vi "WSVCAP SHL FPGA TL Top Level.vi"() -> ()   [LabVIEW 2012]
uses:
  Type Defs/WSVCAP SHL State.ctl
  Type Defs/WSVCAP SHL Transaction Enum.ctl
  Type Defs/WSVCAP SHL Communication Loop State.ctl
  Type Defs/WSVCAP SHL FIFO Operation Enum.ctl
  Type Defs/WSVCAP SHL Operation Step Enum.ctl
  Type Defs/WSVCAP SHL Procedure Step Enum.ctl
  Type Defs/WSVCAP SHL Transaction Step Enum.ctl
  <vilib>/Platform/TimedLoop/XDataNode/timing_clust.ctl
  <vilib>/Platform/TimedLoop/XDataNode/nitl_modes.ctl
  <vilib>/Platform/TimedLoop/XDataNode/wakeup.ctl
  WSVCAP Shell FPGA Low Level/WSVCAP SHL FPGA LL RFFE Debug Global.vi
  WSVCAP Shell FPGA Low Level/WSVCAP SHL FPGA LL SPI Debug Global.vi
  WSVCAP Shell FPGA Low Level/WSVCAP SHL FPGA LL I2C Debug Global.vi
  <vilib>/Platform/TimedLoop/XDataNode/XDataNode.xnode
  <vilib>/Platform/TimedLoop/XDataNode/XDNodeRunTimeDep.lvlib
panel:
  in  "Stop Cycle":bool
  out "Cycle Count":u64
  in  "Socket Mask":u64=1 format="%012x"
  in  "Display CH (1-48)":i32=1 min=1 max=48 step=1
  out "Status":i32
  out "Read Data":u64
  in  "Transaction":T1
  in  "Bytes to Write":u8=8
  in  "Sub Address":u8=1 format="%02x"
  in  "Ack Read Status":bool
  out "Read Status Flag":bool
  in  "Exit":bool
  out "Waveform Chart":cluster{i16, i16, i16, i16}(graph)
  in  "Wait Ticks":u32=20
  in  "Slave Address":u8=1 format="%02x"
  in  "Bytes to Read":u8=8
  in  "Start":bool
  in  "Cmd":T2
  in  "Ack Read":bool
  out "Read Flag":bool
  in  "Write Flag":bool
  in  "Write Data":u64
  # "Control"
  # "I2C Configuration Parameters"
  # "Host Data Transfer"
  # "Command Type"
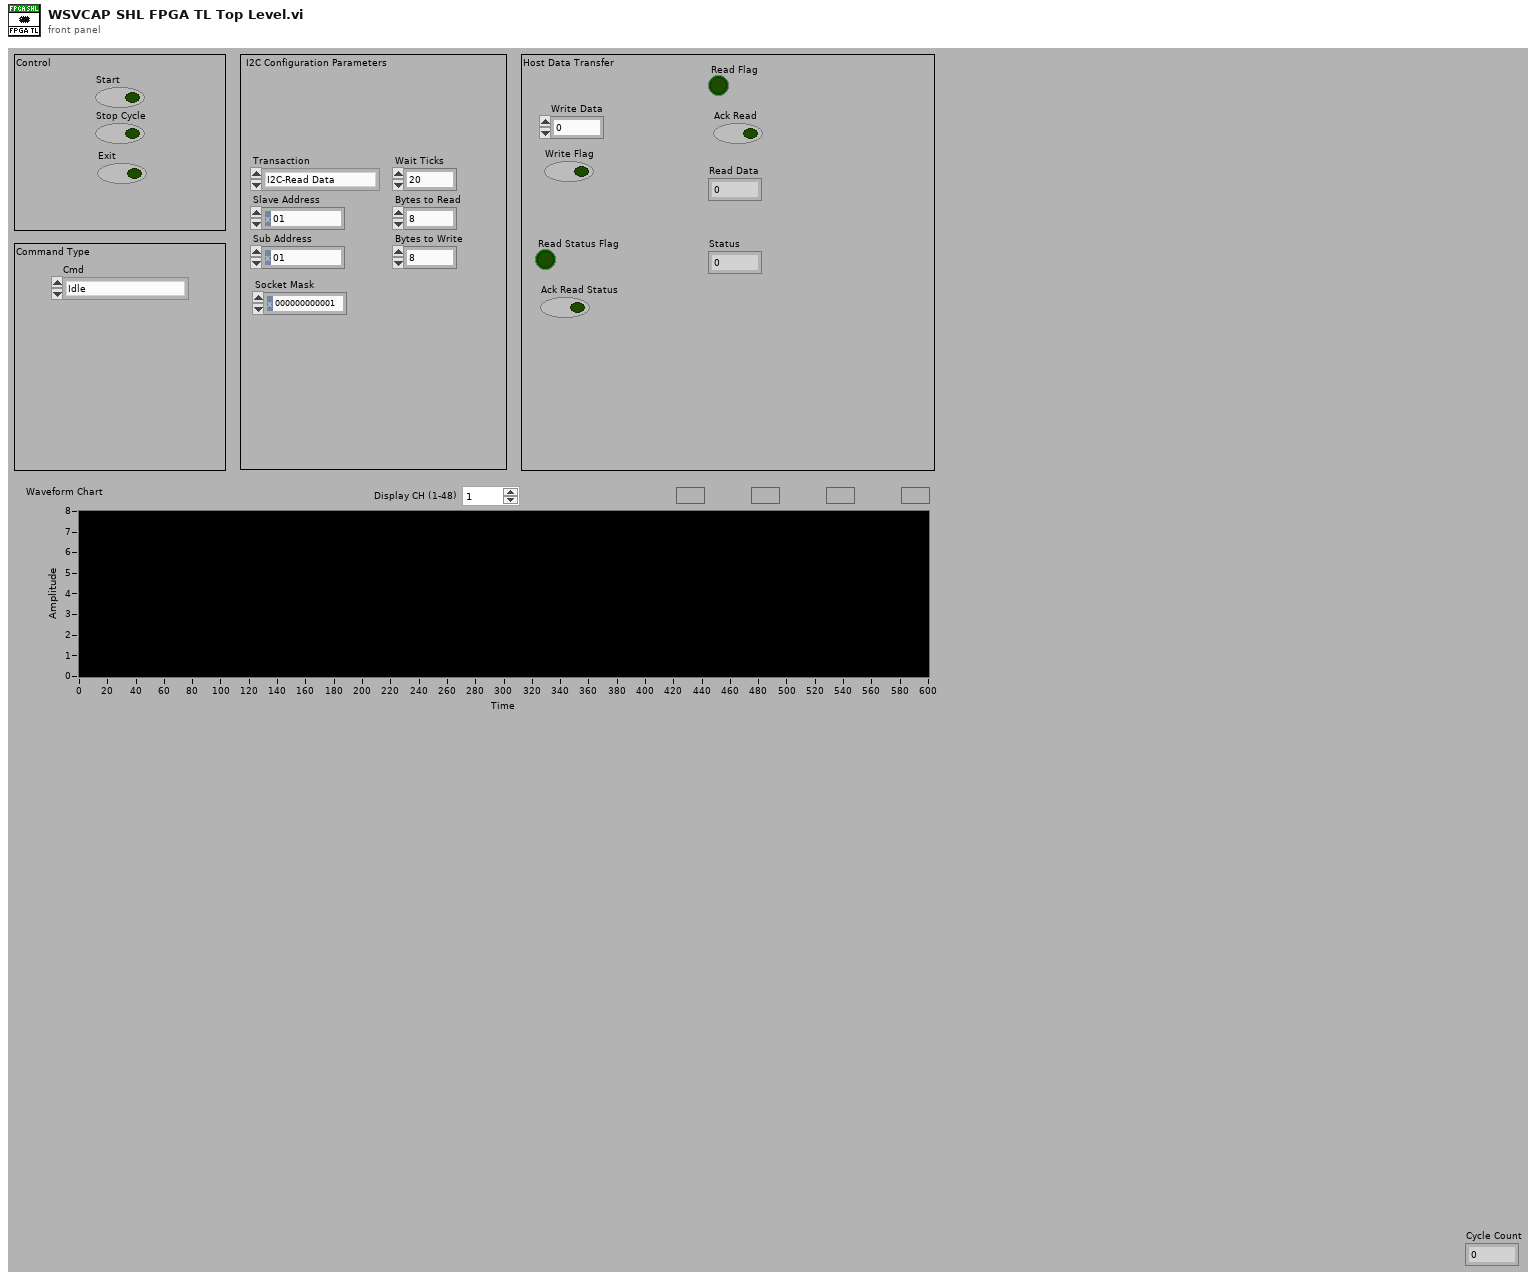
[diagram p1: front panel]
types:
  T1 = typedef "WSVCAP SHL Transaction Enum.ctl" = enum16{"I2C-Read Data", "I2C-Write Data", "SPI-Write/Read Data", "RFFE-Ext Write", "RFFE-Ext Read"}
  T2 = typedef "WSVCAP SHL State.ctl" = enum8{"Idle", "Transfer Data"}
  T3 = typedef "WSVCAP SHL Communication Loop State.ctl" = enum8{"Idle", "Initialize", "Pre-Transmission", "Transmit Data", "Post Transmition", "Operation Complete"}
  T4 = typedef "WSVCAP SHL FIFO Operation Enum.ctl" = enum16{"Create FIFO/Memory", "Get Write FIFO Status", "Get Read FIFO Status", "Put Element in Write", "Put Element in Read", "Get Element from Write", "Get Element from Read"}
  T5 = typedef "WSVCAP SHL Procedure Step Enum.ctl" = enum16{"I2C Start/Stop - 1: Set Clock Low", "I2C Start/Stop - 2: Wait", "I2C Start/Stop - 3: Set Data I", "I2C Start/Stop - 4: Wait", "I2C Start/Stop - 5: Set Clock High", "I2C Start/Stop - 6: Wait", "I2C Start/Stop - 7: Set Data II", "I2C Start/Stop - 8: Wait", "I2C Start/Stop - 9: Set Clock Low", "I2C Start/Stop - 10: Wait", "I2C Read ACK - 1: Set Clock High", "I2C Read ACK - 2: Wait", "I2C Read ACK - 3: Read ACK Bit", "I2C Read ACK - 4: Wait", "I2C Read ACK - 5: Set Clock Low", "I2C Read ACK - 6: Wait", "I2C Write ACK - 1: Write ACK Bit", "I2C Write ACK - 2: Wait", "I2C Write ACK - 3: Set Clock High", "I2C Write ACK - 4: Wait", "I2C Write ACK - 5: Set Clock Low", "I2C Write ACK - 6: Wait", "I2C Write ACK - 7: Set Data Low", "I2C Send Add - 1: Reset Bits Remaining", "I2C Send Add - 2: Set Data Bit", "I2C Send Add - 3: Wait", "I2C Send Add - 4: Set Clock High", "I2C Send Add - 5: Wait", "I2C Send Add - 6: Set Clock Low", "I2C Send Add - 7: Wait", "I2C Send Add - 8: Check Bits Remaining", "I2C Send Data - 1: Reset Bits Remaining", "I2C Send Data - 2: Load Write Bit from FIFO", "I2C Send Data - 3: Set Data Bit", "I2C Send Data - 4: Wait", "I2C Send Data - 5: Set Clock High", "I2C Send Data - 6: Wait", "I2C Send Data - 7: Set Clock Low", "I2C Send Data - 8: Wait", "I2C Send Data - 9: Check Bits Remaining", "I2C Receive Data - 1: Reset Bits Remaining", "I2C Receive Data - 2: Wait", "I2C Receive Data - 3: Set Clock High", "I2C Receive Data - 4: Wait", "I2C Receive Data - 5: Read Data Bit", "I2C Receive Data - 6: Wait", "I2C Receive Data - 7: Set Clock Low", "I2C Receive Data - 8: Wait", "I2C Receive Data - 9: Check Bits Remaining", "SPI Clear Lines - 1:Clear", "SPI Send/Receive - 1: Load SDA - Clock Low", "SPI Send/Receive - 2: Wait", "SPI Send/Receive - 3: Load DATO - Clock High", "SPI Send/Receive - 4: Wait", "SPI Wait CMD Delay - 1:Wait", "RFFE Send SSC - 1:Set Low", "RFFE Send SSC - 2:Wait", "RFFE Send SSC - 3:Set SDA High", "RFFE Send SSC - 4:Wait", "RFFE Send SSC - 5:Set SDA Low", "RFFE Send SSC - 6:Wait", "RFFE Send Data - 1:Set SCL High", "RFFE Send Data - 2:Wait", "RFFE Send Data - 3:Set SCL Low", "RFFE Send Data - 4:Wait", "RFFE Send Data - 5:Set SCL High (P)", "RFFE Send Data - 6:Wait", "RFFE Send Data - 7:Set SCL Low (P)", "RFFE Send Data - 8:Wait", "RFFE Send Data - 9:Set SCL High (BP)", "RFFE Send Data - 10:Wait", "RFFE Send Data - 11:Set SCL Low (BP)", "RFFE Send Data - 12:Wait", "RFFE Receive Data - 1:Set SCL High", "RFFE Receive Data - 2:Wait", "RFFE Receive Data - 3:Set SCL Low", "RFFE Receive Data - 4:Wait", "RFFE Receive Data - 5:Set SCL High (BP)", "RFFE Receive Data - 6:Wait", "RFFE Receive Data - 7:Set SCL Low (BP)", "RFFE Receive Data - 8:Wait", "RFFE Wait CMD Delay - 1:Wait", "RFFE Clear Lines - 1:Clear"}
  T6 = typedef "WSVCAP SHL Operation Step Enum.ctl" = enum16{"I2C Send Slave Add - A: Send Start Sequence", "I2C Send Slave Add - B: Load Address Byte", "I2C Send Slave Add - C: Send Address Byte", "I2C Send Slave Add - D: Read Slave ACK", "I2C Send Sub Add - A: Load Sub Address", "I2C Send Sub Add - B: Send Address Byte", "I2C Send Sub Add - C: Read Slave ACK", "I2C Send Data - A: Get Byte from FIFO", "I2C Send Data - B: Send Data Byte", "I2C Send Data - C: Read Slave ACK", "I2C Send Data - D: Send Stop Sequence", "I2C Read Data - A: Load Bytes to Read", "I2C Read Data - B: Receive Byte", "I2C Read Data - C: Write Master ACK", "I2C Read Data - D: Send Stop Sequence", "SPI Write/Read - A: SPI-Clear Lines", "SPI Write/Read - B: SPI-Send/Receive Data", "SPI Write/Read - C: SPI-Wait CMD Delay", "SPI Write/Read - D:SPI-Clear Lines", "RFFE Read Data - A: Send SSC", "RFFE Read Data - B: Send CMD Frame", "RFFE Read Data - C: Receive Byte", "RFFE Write Data - A: Send SSC", "RFFE Write Data - B: Send Data", "RFFE Write Data - C: Wait CMD Delay", "RFFE Write Data - D: Clear Lines"}
  T7 = typedef "WSVCAP SHL Transaction Step Enum.ctl" = enum16{"I2C Write - I:Send Slave Address", "I2C Write - II:Send Sub Address", "I2C Write - III:Send Data Bytes", "I2C Read - I:Send Slave Address (W)", "I2C Read - II:Send Sub Address", "I2C Read - III:Send Slave Address (R)", "I2C Read - IV:Read Data Bytes", "SPI Write/Read - I:SPI-Write/Read Data", "RFFE Ext Write - I.Write Data", "RFFE Ext Read - I:Read Data"}
  T8 = typedef "XDNodeRunTimeDep.lvlib/timing_clust.ctl" = cluster{"Expected End [f-1]":u64, "Actual End [f-1]":u64, "Finished Late? [f-1]":bool, "Expected End [i-1]":u64, "Actual End [i-1]":u64, "Finished Late? [i-1]":bool, "Expected Start [i]":u64, "Actual Start [i]":u64, "Expected Start [f]":u64, "Actual Start [f]":u64, "Source Name":string, "Structure Name":string, "Period":i64, "Deadline":i64, "Offset":i64, "Start":i64, "Priority":i32, "Timeout":i32, "Mode":T9, "Wakeup Reason":T10, "Error":errorcluster, "Source Type":string, "Secondary Source Type":string, "Global End Time":u64, "Global Start Time":u64, "Frame Duration":u64, "Iteration Duration":u64, "Assigned CPU":i32, "I/O Scan Engine Mode":u32}
  T9 = typedef "XDNodeRunTimeDep.lvlib/nitl_modes.ctl" = enum32{"No Change", "Process missed periods, maintain original phase", "Discard missed periods, maintain original phase", "Process missed periods, ignore original phase", "Discard missed periods, ignore original phase"}
  T10 = typedef "XDNodeRunTimeDep.lvlib/wakeup.ctl" = enum32{"Normal", "Aborted", "Asynchronous wakeup", "Timing source error", "Timed loop error", "Timeout"}
  T11 = typedef "WSVCAP SHL Transaction Cluster.ctl" = cluster{"Transaction":T1, "Write Byte":u8, "Write Bits Remaining":u8, "Read Bits Remaining":u8, "Read Bytes Remaining":u8, "Wait Ticks Remaining":u32, "Slave Address":u8, "Bytes to Read":u8, "Bytes to Write":u8, "Sub Address":u8, "Socket Mask":u64, "Write CMD [1-4]":u8, "Write Bit Index [0-39]":u8, "CMD Delay (Ticks)":u32, "Commands per Cycle [1-4]":u8, "CMD Length [1-48]":u8, "Cycle Count":u64, "Cycle Mode":bool, "CMD 1 Length (Bits)":u8, "CMD 2 Length (Bits)":u8, "CMD 3 Length (Bits)":u8, "CMD 4 Length (Bits)":u8, "CMD 1 Delay (Ticks)":u32, "CMD 2 Delay (Ticks)":u32, "CMD 3 Delay (Ticks)":u32, "CMD 4 Delay (Ticks)":u32, "CMD 1":u64, "CMD 2":u64, "CMD 3":u64, "CMD 4":u64, "Cycle CMD":u64, "Transaction Step":T7, "Operation Step":T6, "Procedure Step":T5, "Start Operation":bool, "Start Procedure":bool, "Procedure":T12, "Wait Ticks":u32}
  T12 = typedef "WSVCAP SHL Procedure Enum.ctl" = enum16{"None", "I2C-Send Start/Stop Sequence", "I2C-Send Address Byte", "I2C-Send Data Byte", "I2C-Read ACK", "I2C-Receive Byte", "I2C-Write ACK", "SPI-Clear Lines", "SPI-Send/Receive", "SPI-Wait CMD Delay", "RFFE-Clear Lines", "RFFE-Send SSC", "RFFE-Send Data", "RFFE-Receive Data", "RFFE-Wait CMD Delay"}
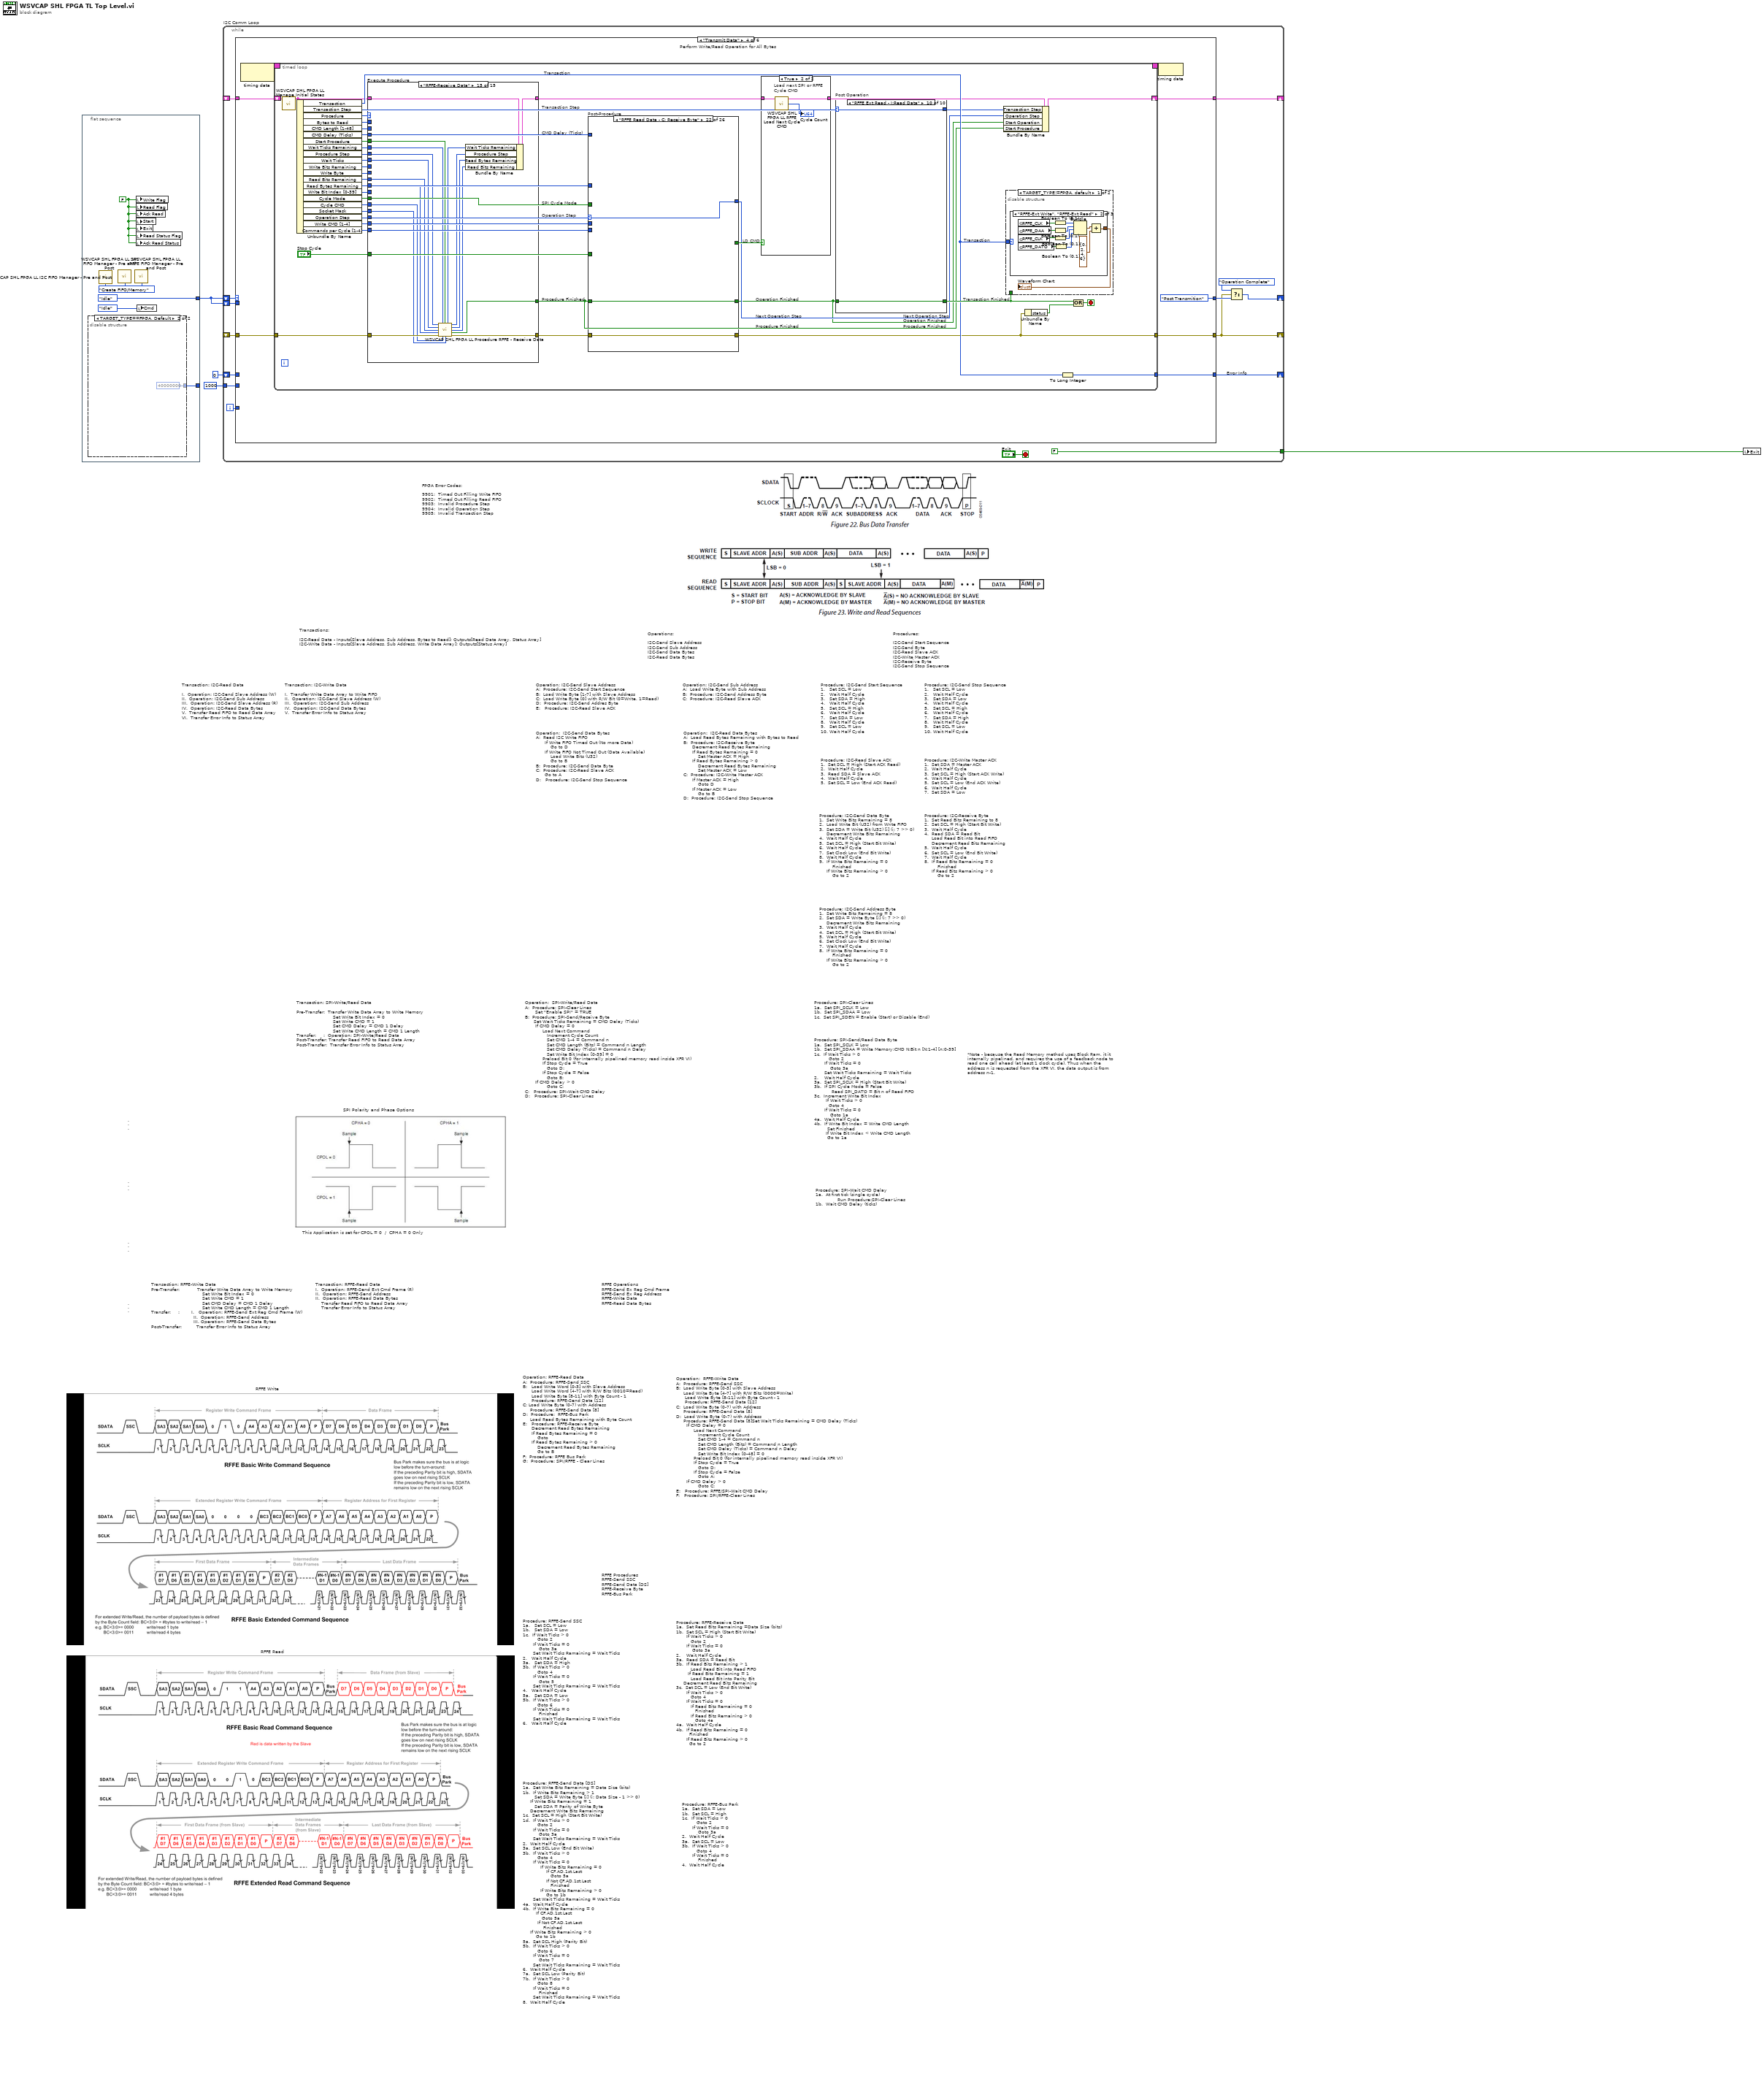
[diagram p0: block diagram]
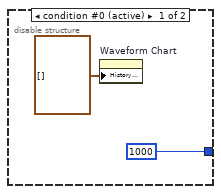
[diagram p2: hidden frame]
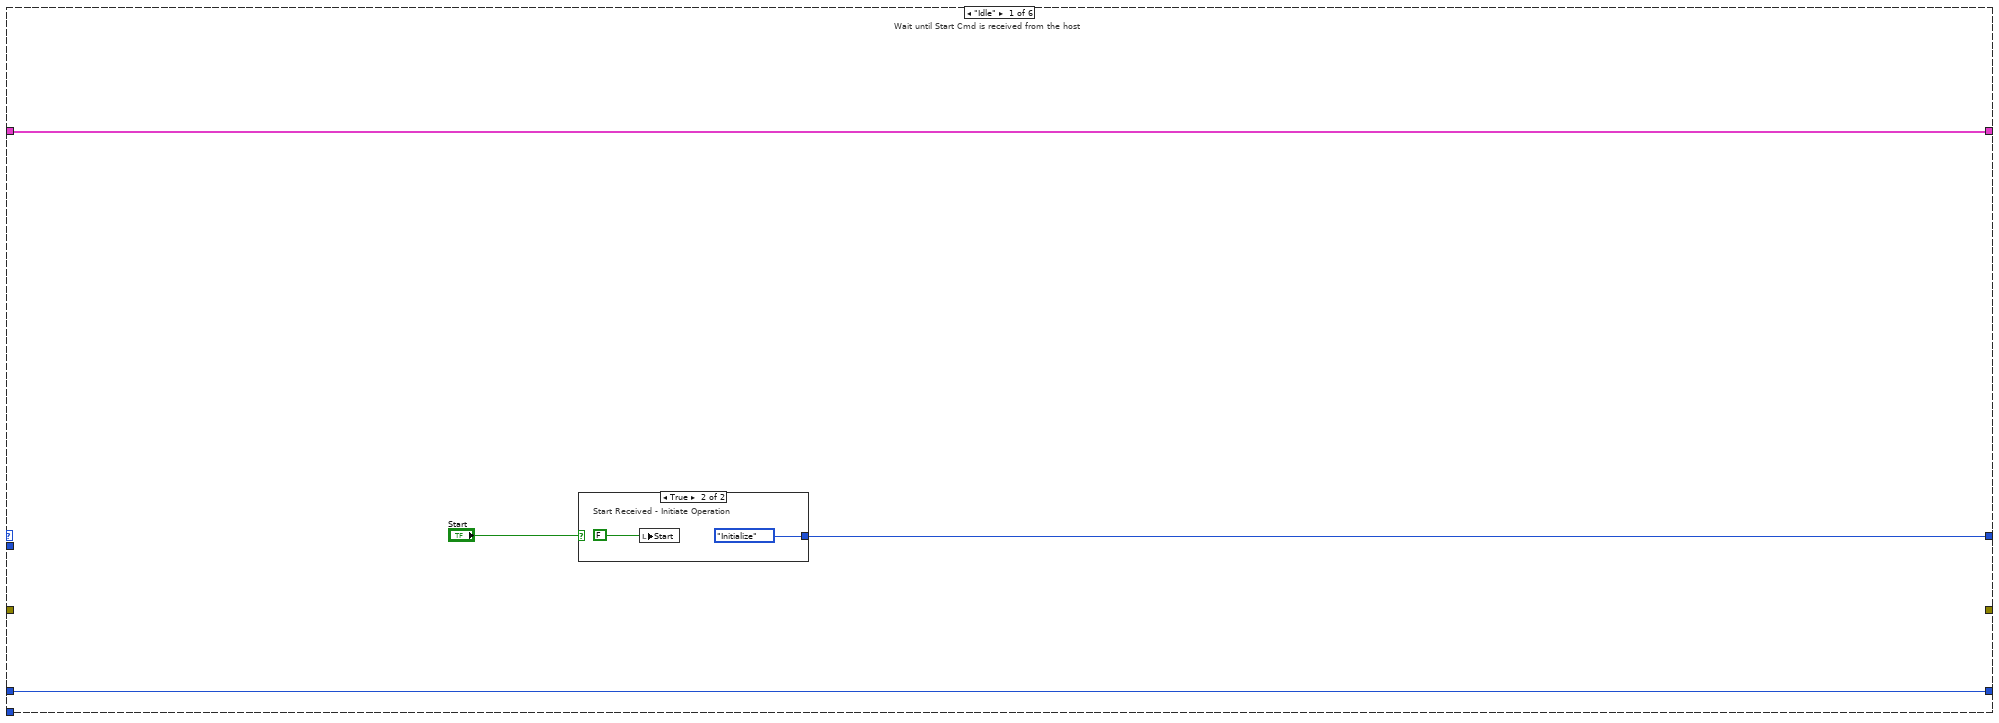
[diagram p3: hidden frame]
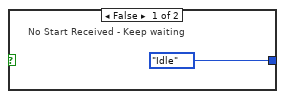
[diagram p4: hidden frame]
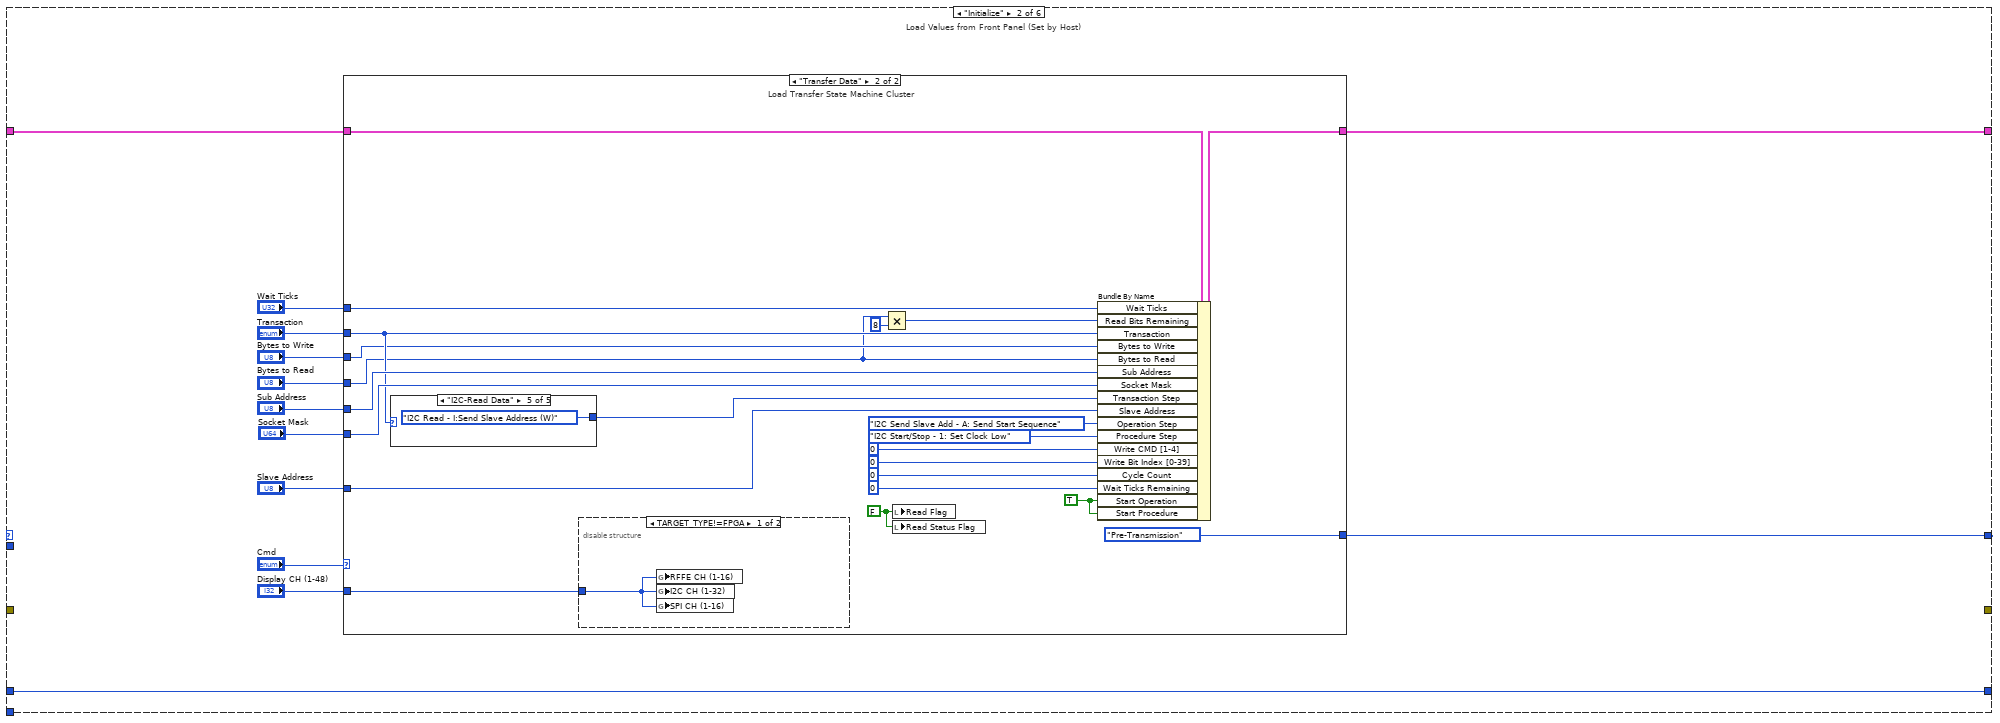
[diagram p5: hidden frame]
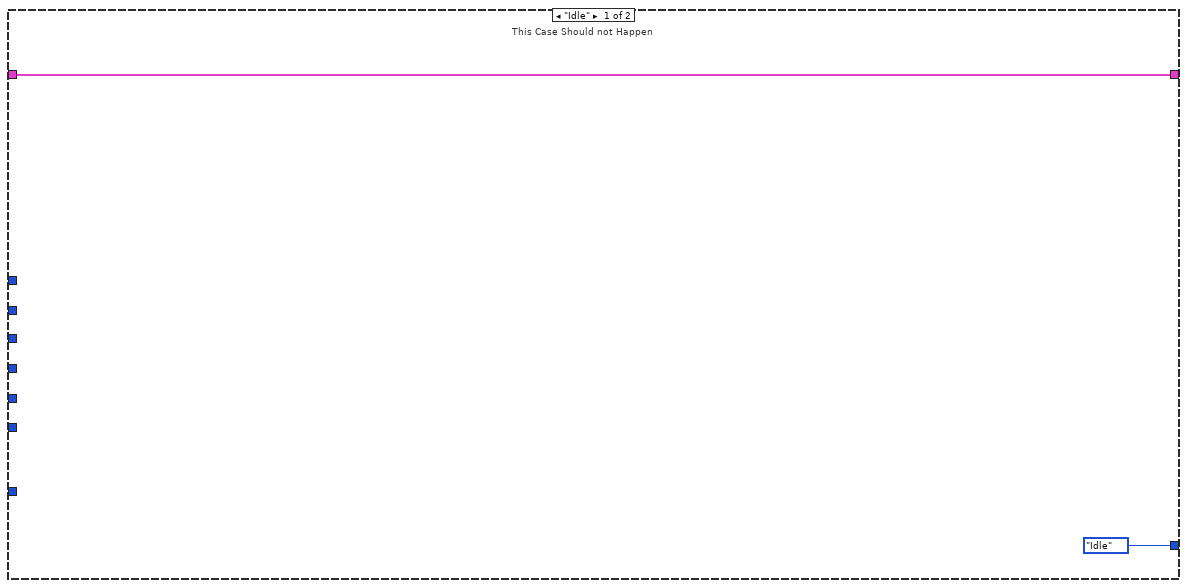
[diagram p6: hidden frame]
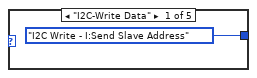
[diagram p7: hidden frame]
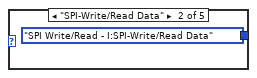
[diagram p8: hidden frame]
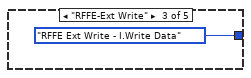
[diagram p9: hidden frame]
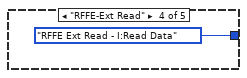
[diagram p10: hidden frame]
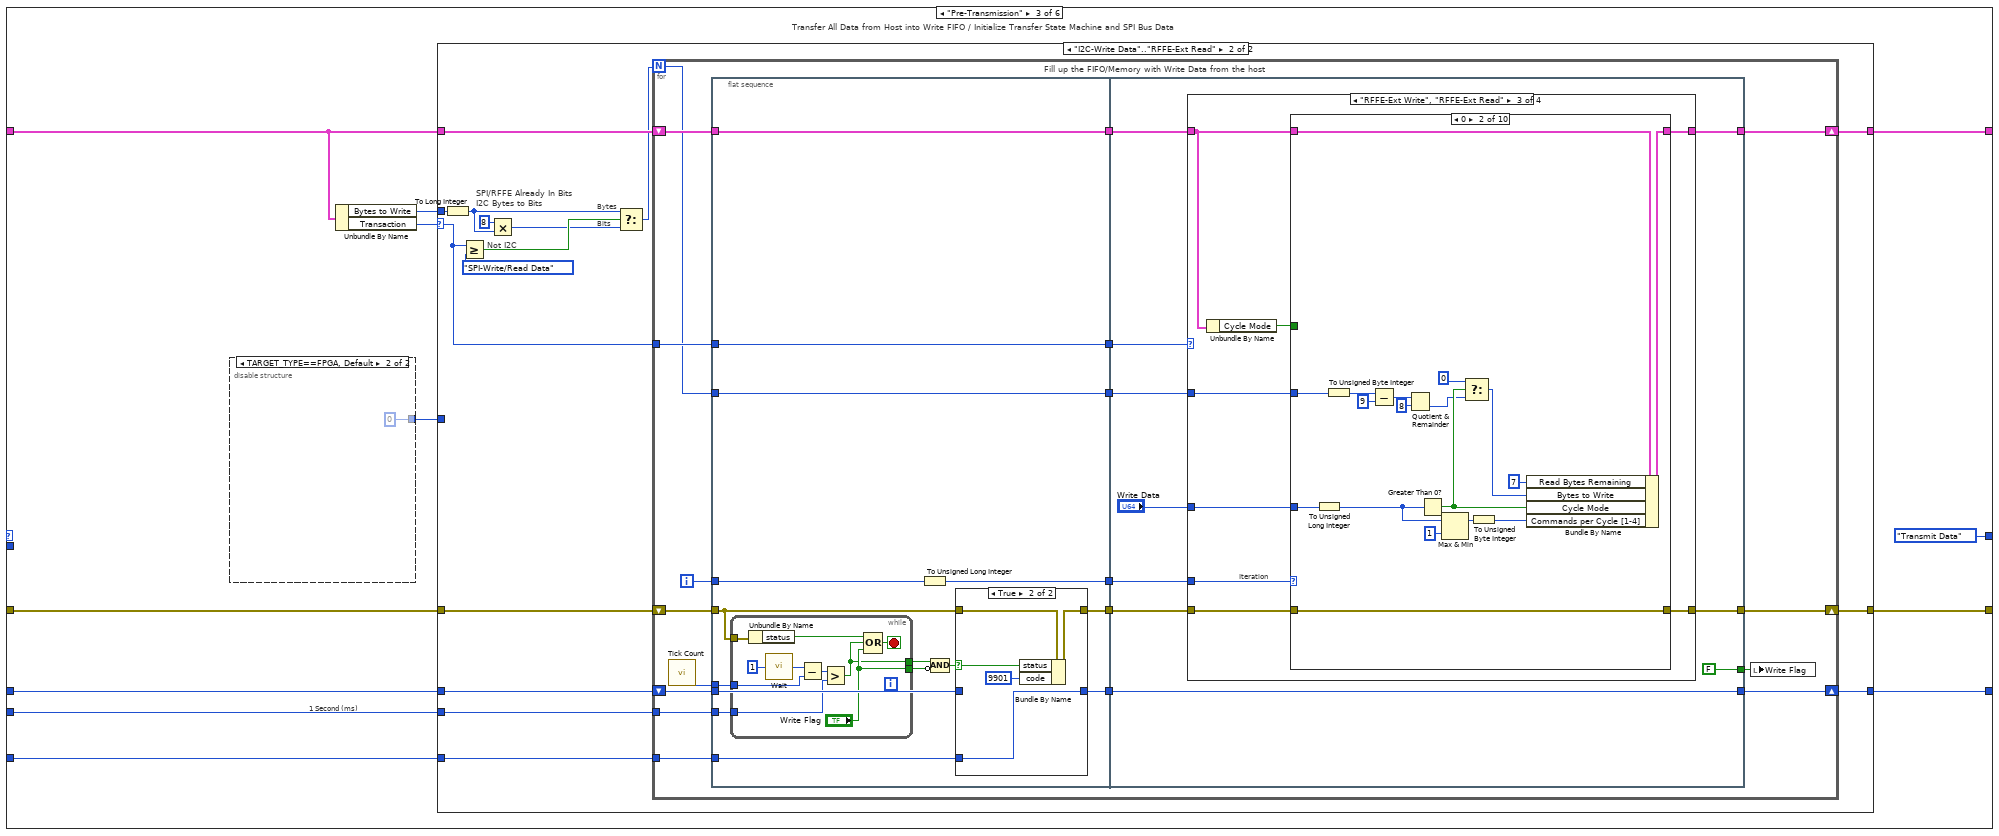
[diagram p12: hidden frame]
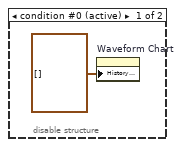
[diagram p13: hidden frame]
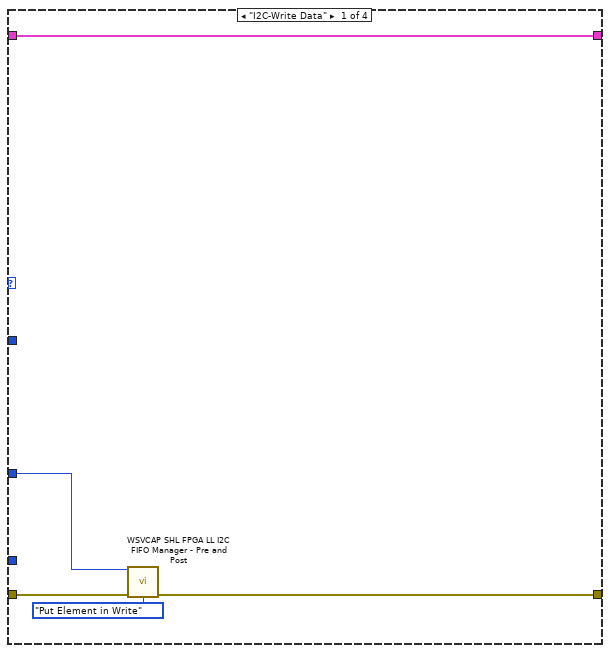
[diagram p16: hidden frame]
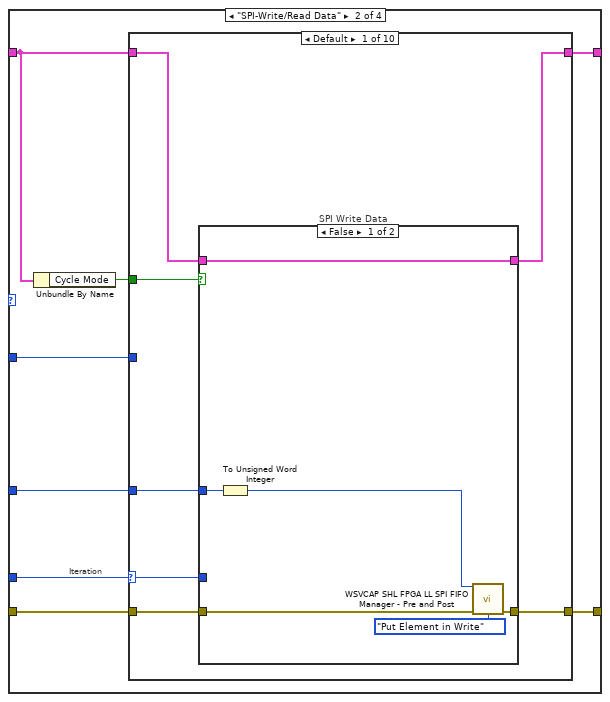
[diagram p17: hidden frame]
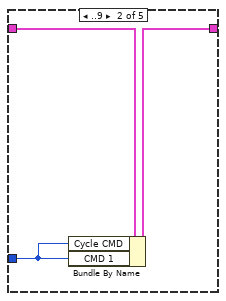
[diagram p19: hidden frame]
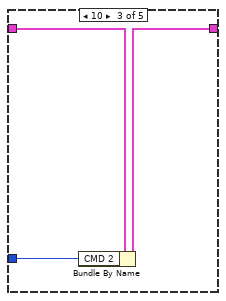
[diagram p20: hidden frame]
diagram:
  # "Operation:  RFFE-Write Data\nA:  Procedure: RFFE-Send SSC\nB:  Load Write Byte [0-3] with Slave Address\n     Load Write Byte [4-7] with R/W Bits (0000=Write)\n      Load Write Byte [8-11] with Byte Count - 1\n      Procedure: RFFE-Send Data [12]\nC:  Load Write Byte (0-7) with Address\n     Procedure: RFFE-Send Data [8]\nD:  Load Write Byte (0-7) with Address\n     Procedure: RFFE-Send Data [8]Set Wait Ticks Remaining = CMD Delay (Ticks)\n       If CMD Delay = 0\n            Load Next Command\n               Increment Cycle Count\n               Set CMD 1-4 = Command n\n               Set CMD Length (Bits) = Command n Length\n               Set CMD Delay (Ticks) = Command n Delay\n               Set Write Bit Index [0-48] = 0\n            Preload Bit 0 (for internally pipelined memory read inside XFR VI)\n            If Stop Cycle = True\n               Goto D:\n            If Stop Cycle = False\n               Goto A:\n       If CMD Delay > 0\n               Goto C:\nE:   Procedure: RFFE/SPI-Wait CMD Delay          \nF:   Procedure: SPI/RFFE-Clear Lines"
  # "Operation: RFFE-Read Data\nA:  Procedure: RFFE-Send SSC\nB:   Load Write Word [0-3] with Slave Address\n      Load Write Word [4-7] with R/W Bits (0010=Read)\n      Load Write Byte [8-11] with Byte Count - 1\n      Procedure: RFFE-Send Data [12]\nC: Load Write Byte (0-7) with Address\n     Procedure: RFFE-Send Data [8]\nD:  Procedure:  RFFE-Bus Park\n     Load Read Bytes Remaining with Byte Count\nE:   Procedure: RFFE-Receive Byte\n      Decrement Read Bytes Remaining\n      If Read Bytes Remaining = 0\n          Goto\n      If Read Bytes Remaining > 0\n          Decrement Read Bytes Remaining\n          Go to B\nF:  Procedure: RFFE Bus Park\nG:  Procedure: SPI/RFFE - Clear Lines"
  # "RFFE Write"
  # "RFFE Read"
  # "Transaction: RFFE-Write Data\nPre-Transfer:            Transfer Write Data Array to Write Memory\n                                   Set Write Bit Index = 0\n                                   Set Write CMD = 1\n                                   Set CMD Delay = CMD 1 Delay\n                                   Set Write CMD Length = CMD 1 Length\nTransfer:     :        I.   Operation: RFFE-Send Ext Reg Cmd Frame (W)\n                             II.  Operation: RFFE-Send Address\n                             III. Operation: RFFE-Send Data Bytes\nPost-Transfer:          Transfer Error Info to Status Array"
  # "Procedure: RFFE-Send Data [DS]\n1a.  Set Write Bits Remaining = Data Size (bits)\n1b.  If Write Bits Remaining > 1\n        Set SDA = Write Byte [i] (i: Data Size - 1 >> 0)\n     If Write Bits Remaining = 1\n        Set SDA = Parity of Write Byte\n     Decrement Write Bits Remaining\n1c.  Set SCL = High (Start Bit Write)\n1d.  If Wait Ticks > 0\n          Goto 2\n       If Wait Ticks = 0 \n           Goto 3a\n       Set Wait Ticks Ramaining = Wait Ticks\n2.  Wait Half Cycle\n3a.  Set SCL Low (End Bit Write)\n3b.  If Wait Ticks > 0\n          Goto 4\n       If Wait Ticks = 0 \n            If Write Bits Remaining = 0\n                If CF,AD,1st,Last\n                   Goto 5a\n                If Not CF,AD,1st,Last\n                   Finished\n            If Write Bits Remaining > 0\n                Go to 1b\n       Set Wait Ticks Ramaining = Wait Ticks\n4a.  Wait Half Cycle\n4b.  If Write Bits Remaining = 0\n         If CF,AD,1st,Last\n             Goto 5a\n          If Not CF,AD,1st,Last\n              Finished\n     If Write Bits Remaining > 0\n         Go to 1b\n5a.  Set SCL High (Parity Bit)\n5b.  If Wait Ticks > 0\n          Goto 6\n       If Wait Ticks = 0 \n           Goto 7\n       Set Wait Ticks Ramaining = Wait Ticks\n6.  Wait Half Cycle\n7a.  Set SCL Low (Parity Bit)\n7b.  If Wait Ticks > 0\n          Goto 8\n       If Wait Ticks = 0 \n           Finished\n       Set Wait Ticks Ramaining = Wait Ticks\n8.  Wait Half Cycle"
  # "Procedure: RFFE-Bus Park\n1a.  Set SDA = Low\n1b.  Set SCL = High\n1c.  If Wait Ticks > 0\n          Goto 2\n       If Wait Ticks = 0 \n           Goto 3a\n2.  Wait Half Cycle\n3a.  Set SCL = Low\n3b.  If Wait Ticks > 0\n          Goto 4\n       If Wait Ticks = 0 \n           Finished\n4.  Wait Half Cycle"
  # "Procedure: RFFE-Send SSC\n1a.   Set SCL = Low\n1b.   Set SDA = Low\n1c.  If Wait Ticks > 0\n          Goto 2\n       If Wait Ticks = 0 \n           Goto 3a\n       Set Wait Ticks Ramaining = Wait Ticks\n2.   Wait Half Cycle\n3a.   Set SDA = High\n3b.  If Wait Ticks > 0\n          Goto 4\n       If Wait Ticks = 0 \n           Goto 5\n       Set Wait Ticks Ramaining = Wait Ticks\n4.   Wait Half Cycle\n5a.   Set SDA = Low\n5b.  If Wait Ticks > 0\n          Goto 6\n       If Wait Ticks = 0 \n           Finished\n       Set Wait Ticks Ramaining = Wait Ticks\n6.   Wait Half Cycle"
  # "Procedure: RFFE-Receive Data\n1a.  Set Read Bits Remaining =Data Size (bits)\n1b.  Set SCL = High (Start Bit Write)\n       If Wait Ticks > 0\n          Goto 2\n       If Wait Ticks = 0 \n           Goto 3a\n2.    Wait Half Cycle\n3a.  Read SDA = Read Bit\n3b.  If Read Bits Remaining > 1\n          Load Read Bit into Read FIFO\n        If Read Bits Remaining = 1\n          Load Read Bit into Parity Bit\n     Decrement Read Bits Remaining\n3c.  Set SCL = Low (End Bit Write)\n       If Wait Ticks > 0\n          Goto 4\n       If Wait Ticks = 0\n          If Read Bits Remaining = 0\n             Finished\n          If Read Bits Remaining > 0\n             Goto 4a\n4a.  Wait Half Cycle\n4b.  If Read Bits Remaining = 0\n         Finished\n       If Read Bits Remaining > 0\n         Go to 2"
  # "RFFE Procedures\nRFFE-Send SSC\nRFFE-Send Data [DS]\nRFFE-Receive Byte\nRFFE-Bus Park"
  # "Transaction: RFFE-Read Data\nI.  Operation: RFFE-Send Ext Cmd Frame (R)\nII.  Operation: RFFE-Send Address\nII.  Operation: RFFE-Read Data Bytes\n    Transfer Read FIFO to Read Data Array\n    Transfer Error Info to Status Array"
  # "RFFE Operations\nRFFE-Send Ex Reg Cmd Frame\nRFFE-Send Ex Reg Address\nRFFE-Write Data\nRFFE-Read Data Bytes"
  # "*Note - because the Read Memory method uses Block Ram, it it internally pipelined, and requires the use of a feedback node to read one call ahead (at least 1 clock cycle). Thus when the address n is requested from the XFR VI, the data output is from address n-1."
  # "SPI Polarity and Phase Options"
  # "Procedure: SPI-Wait CMD Delay\n1a.  At first tick (single cycle)\n               Run Procedure:SPI-Clear Lines\n1b.  Wait CMD Delay (ticks)"
  # "Procedure: SPI-Clear Lines\n1a.  Set SPI_SCLK = Low\n1b.  Set SPI_SDAA = Low\n1c.  Set SPI_SDEN = Enable (Start) or Disable (End)"
  # "This Application is set for CPOL = 0  /  CPHA = 0 Only"
  # "Procedure: SPI-Send/Read Data Byte\n1a.  Set SPI_SCLK = Low\n1b.  Set SPI_SDAA = Write Memory:CMD N:Bit n [N:1-4] [n:0-39] \n1c.  If Wait Ticks > 0\n          Goto 2\n       If Wait Ticks = 0 \n           Goto 3a\n       Set Wait Ticks Ramaining = Wait Ticks\n2.    Wait Half Cycle\n3a.  Set SPI_SCLK = High (Start Bit Write)\n3b.  If SPI Cycle Mode = False\n            Read SPI_DATO = Bit n of Read FIFO            \n3c.  Increment Write Bit Index\n        If Wait Ticks > 0\n          Goto 4\n       If Wait Ticks = 0 \n           Goto 1a \n4a.  Wait Half Cycle\n4b.  If Write Bit Index = Write CMD Length\n         Set Finished\n        If Write Bit Index < Write CMD Length\n         Go to 1a"
  # ".\n.\n."
  # ".\n.\n."
  # ".\n.\n."
  # ".\n.\n."
  # "Operation:  SPI-Write/Read Data\nA:  Procedure: SPI-Clear Lines\n       Set \"Enable SPI\" = TRUE \nB:  Procedure: SPI-Send/Receive Byte\n      Set Wait Ticks Remaining = CMD Delay (Ticks)\n       If CMD Delay = 0\n            Load Next Command\n               Increment Cycle Count\n               Set CMD 1-4 = Command n\n               Set CMD Length (Bits) = Command n Length\n               Set CMD Delay (Ticks) = Command n Delay\n               Set Write Bit Index [0-39] = 0\n            Preload Bit 0 (for internally pipelined memory read inside XFR VI)\n            If Stop Cycle = True\n               Goto D:\n            If Stop Cycle = False\n               Goto B:\n       If CMD Delay > 0\n               Goto C:\nC:   Procedure: SPI-Wait CMD Delay          \nD:   Procedure: SPI-Clear Lines"
  # "FPGA Error Codes:\n\n9901:  Timed Out Filling Write FIFO\n9902:  Timed Out Filling Read FIFO\n9903:  Invalid Procedure Step\n9904:  Invalid Operation Step\n9905:  Invalid Transaction Step"
  # "Transaction: SPI-Write/Read Data\n\nPre-Transfer:  Transfer Write Data Array to Write Memory\n                         Set Write Bit Index = 0\n                         Set Write CMD = 1\n                         Set CMD Delay = CMD 1 Delay\n                         Set Write CMD Length = CMD 1 Length\nTransfer:     :  Operation: SPI-Write/Read Data\nPost-Transfer: Transfer Read FIFO to Read Data Array\nPost-Transfer:  Transfer Error Info to Status Array"
  # "Procedure: I2C-Send Address Byte\n1.  Set Write Bits Remaining = 8\n2.  Set SDA = Write Byte [i] (i: 7 >> 0)\n     Decrement Write Bits Remaining\n3.  Wait Half Cycle\n4.  Set SCL = High (Start Bit Write)\n5.  Wait Half Cycle\n6.  Set Clock Low (End Bit Write)\n7.  Wait Half Cycle\n8.  If Write Bits Remaining = 0\n         Finished\n     If Write Bits Remaining > 0\n         Go to 2"
  # "Procedure: I2C-Write Master ACK\n1.  Set SDA = Master ACK\n2.  Wait Half Cycle\n3.  Set SCL = High (Start ACK Write)\n4.  Wait Half Cycle\n5.  Set SCL = Low (End ACK Write)\n6.  Wait Half Cycle\n7.  Set SDA = Low"
  # "Procedure: I2C-Send Start Sequence\n1.   Set SCL = Low\n2.   Wait Half Cycle\n3.   Set SDA = High\n4.   Wait Half Cycle\n5.   Set SCL = High\n6.   Wait Half Cycle\n7.   Set SDA = Low\n8.   Wait Half Cycle\n9.   Set SCL = Low\n10. Wait Half Cycle"
  # "Procedure: I2C-Send Stop Sequence\n1.   Set SCL = Low\n2.   Wait Half Cycle\n3.   Set SDA = Low\n4.   Wait Half Cycle\n5.   Set SCL = High\n6.   Wait Half Cycle\n7.   Set SDA = High\n8.   Wait Half Cycle\n9.   Set SCL = Low\n10. Wait Half Cycle"
  # "Procedure: I2C-Read Slave ACK\n1.  Set SCL = High (Start ACK Read)\n2.  Wait Half Cycle\n3.  Read SDA = Slave ACK\n4.  Wait Half Cycle\n5.  Set SCL = Low (End ACK Read)"
  # "Procedure: I2C-Receive Byte\n1.  Set Read Bits Remaining to 8\n2.  Set SCL = High (Start Bit Write)\n3.  Wait Half Cycle\n4.  Read SDA = Read Bit\n     Load Read Bit into Read FIFO\n     Decrement Read Bits Remaining\n5.  Wait Half Cycle\n6.  Set SCL = Low (End Bit Write)\n7.  Wait Half Cycle\n8.  If Read Bits Remaining = 0\n         Finished\n     If Read Bits Remaining > 0\n         Go to 2"
  # "Procedure: I2C-Send Data Byte\n1.  Set Write Bits Remaining = 8\n2.  Load Write Bit (U32) from Write FIFO\n3.  Set SDA = Write Bit (U32) [i] (i: 7 >> 0)\n     Decrement Write Bits Remaining\n4.  Wait Half Cycle\n5.  Set SCL = High (Start Bit Write)\n6.  Wait Half Cycle\n7.  Set Clock Low (End Bit Write)\n8.  Wait Half Cycle\n9.  If Write Bits Remaining = 0\n         Finished\n     If Write Bits Remaining > 0\n         Go to 2"
  # "Operation:  I2C-Read Data Bytes\nA:  Load Read Bytes Remaining with Bytes to Read\nB:  Procedure: I2C-Receive Byte\n      Decrement Read Bytes Remaining\n      If Read Bytes Remaining = 0\n          Set Master ACK = High\n      If Read Bytes Remaining > 0\n          Decrement Read Bytes Remaining\n          Set Master ACK = Low\nC:  Procedure: I2C-Write Master ACK\n      If Master ACK = High\n          Goto D\n      If Master ACK = Low\n          Go to B\nD:  Procedure: I2C-Send Stop Sequence"
  # "Operation:  I2C-Send Data Bytes\nA:  Read I2C Write FIFO\n      If Write FIFO Timed Out (No more Data)\n          Go to D\n      If Write FIFO Not Timed Out (Data Available)\n          Load Write Bits (U32)\n          Go to B\nB:  Procedure: I2C-Send Data Byte\nC:  Procedure: I2C-Read Slave ACK\n      Go to A\nD:   Procedure: I2C-Send Stop Sequence"
  # "Operation: I2C-Send Sub Address\nA:  Load Write Byte with Sub Address\nB:  Procedure: I2C-Send Address Byte\nC:  Procedure: I2C-Read Slave ACK"
  # "Procedures:\n\nI2C-Send Start Sequence\nI2C-Send Byte\nI2C-Read Slave ACK\nI2C-Write Master ACK\nI2C-Receive Byte\nI2C-Send Stop Sequence"
  # "Transaction: I2C-Write Data\n\nI.  Transfer Write Data Array to Write FIFO\nII.  Operation: I2C-Send Slave Address (W)\nIII.  Operation: I2C-Send Sub Address\nIV.  Operation: I2C-Send Data Bytes\nV.  Transfer Error Info to Status Array"
  # "Transaction: I2C-Read Data\n\nI.  Operation: I2C-Send Slave Address (W)\nII.  Operation: I2C-Send Sub Address\nIII.  Operation: I2C-Send Slave Address (R)\nIV.  Operation: I2C-Read Data Bytes\nV.  Transfer Read FIFO to Read Data Array\nVI.  Transfer Error Info to Status Array"
  # "Transactions:\n\nI2C-Read Data - Inputs[Slave Address, Sub Address, Bytes to Read]; Outputs[Read Data Array, Status Array]\nI2C-Write Data - Inputs[Slave Address, Sub Address, Write Data Array]; Outputs[Status Array]"
  # "Operations:\n\nI2C-Send Slave Address\nI2C-Send Sub Address\nI2C-Send Data Bytes\nI2C-Read Data Bytes"
  # "Operation: I2C-Send Slave Address\nA:  Procedure: I2C-Send Start Sequence\nB:  Load Write Byte [1-7] with Slave Address\nC:  Load Write Byte [0] with R/W Bit (0=Write, 1=Read)\nD:  Procedure: I2C-Send Addres Byte\nE:   Procedure: I2C-Read Slave ACK"
  n1 = flat-sequence {
    tunnel: [WSVCAP_SHL_Communication_Loop_State."Idle" ("Action")] -> w3
    tunnel: [w6] -> _
    frame #0 {
      w5 = WSVCAP_SHL_FIFO_Operation_Enum."Create FIFO/Memory" ("Operation")
      w7 = FALSE ("Done")
      n2 = disable-structure shown="TARGET_TYPE==FPGA, Default" {
        disable-tunnel: [u32 1000 ("x-y") u32 40000000 ("x-y")] -> w6
        frame condition #0 (active) {
          n3 = property on="Waveform Chart" class="WFChart (strict)"("History Data"=cluster{i16, i16, i16, i16}[] []) -> ()  [unwired: 2 in, 2 out]
        }
        frame condition #1 {
        }
      }
      n4 = call "WSVCAP SHL FPGA LL I2C FIFO Manager - Pre and Post.vi"("Operation"=w5) -> ()  [unwired: 12 in, 3 out]
      n5 = call "WSVCAP SHL FPGA LL SPI FIFO Manager - Pre and Post.vi"("Operation"=w5) -> ()  [unwired: 12 in, 3 out]
      n6 = call "WSVCAP SHL FPGA LL RFFE FIFO Manager - Pre and Post.vi"("Operation"=w5) -> ()  [unwired: 12 in, 3 out]
      n7 = local write "Write Flag"(w7) -> ()
      n8 = local write "Read Flag"(w7) -> ()
      n9 = local write "Ack Read"(w7) -> ()
      n10 = local write "Start"(w7) -> ()
      n11 = local write "Exit"(w7) -> ()
      n12 = local write "Read Status Flag"(w7) -> ()
      n13 = local write "Ack Read Status"(w7) -> ()
      n14 = local write "Cmd"(WSVCAP_SHL_State."Idle" ("SPI_CMD_DBG")) -> ()
    }
  }
  n15 = while "I2C Comm Loop" {
    shift-right: [w20] -> _
    shift-left: w3 -> [w27]
    shift-right: [w25] -> _
    shift-left: _ -> [w26]
    tunnel: [FALSE] -> w4
    shift-right: [w19] -> _
    shift-left: _ -> [w22]
    shift-left: w3 -> [w17]
    shift-right: [w16] -> _
    shift-left: 0 -> [w15]
    tunnel: u32 1000 ("x-y") -> [w14]
    i -> [w13]
    stop <- "Exit" stop-if-true
    # "Error Info"
    n16 = case shown="\"Transmit Data\"" w27 {
      tunnel: [w31 w46 WSVCAP_SHL_Communication_Loop_State."Transmit Data" ("Action") WSVCAP_SHL_Communication_Loop_State."Post Transmition" ("Action") WSVCAP_SHL_Communication_Loop_State."Operation Complete" ("Action") WSVCAP_SHL_Communication_Loop_State."Idle" ("Action")] -> w21
      tunnel: w26 -> [w28 w45 w80 w377 w862 w953]
      tunnel: [w28 w44 w79 w376 w862 w953] -> w25
      tunnel: [_ _ w82 w374 w864 _] -> w19
      tunnel: w22 -> [_ _ w87 w375 w865 w958]
      tunnel: w17 -> [_ _ _ _ _ w957]
      tunnel: [w29 w43 w83 w373 w860 _] -> w16
      tunnel: w15 -> [w29 w43 w84 _ w859 w955]
      tunnel: w14 -> [_ _ w86 _ w861 w954]
      tunnel: w13 -> [_ _ w85 _ _ _]
      frame "Idle" {
        # "Wait until Start Cmd is received from the host"
        n17 = case shown="True" "Start" {
          tunnel: [WSVCAP_SHL_Communication_Loop_State."Idle" ("Action") WSVCAP_SHL_Communication_Loop_State."Initialize" ("Action")] -> w31
          frame False {
            # "No Start Received - Keep waiting"
          }
          frame True {
            # "Start Received - Initiate Operation"
            n18 = local write "Start"(FALSE ("SPI_Start")) -> ()
          }
        }
      }
      frame "Initialize" {
        # "Load Values from Front Panel (Set by Host)"
        n19 = case shown="\"Transfer Data\"" "Cmd" {
          tunnel: [WSVCAP_SHL_Communication_Loop_State."Idle" ("Action") WSVCAP_SHL_Communication_Loop_State."Pre-Transmission" ("Action")] -> w46
          tunnel: w45 -> [w48 w69]
          tunnel: [w48 w70] -> w44
          tunnel: "Wait Ticks" -> [_ w56]
          tunnel: "Slave Address" -> [_ w54]
          tunnel: "Sub Address" -> [_ w68]
          tunnel: "Display CH (1-48)" -> [_ w66]
          tunnel: "Transaction" -> [_ w59]
          tunnel: "Bytes to Write" -> [_ w55]
          tunnel: "Bytes to Read" -> [_ w52]
          tunnel: "Socket Mask" -> [_ w67]
          frame "Idle" {
            # "This Case Should not Happen"
          }
          frame "Transfer Data" {
            w53 = FALSE ("Read Flag")
            w57 = TRUE ("Read Flag")
            # "Load Transfer State Machine Cluster"
            n20 = case shown="\"I2C-Read Data\"" w59 {
              tunnel: [WSVCAP_SHL_Transaction_Step_Enum."I2C Write - I:Send Slave Address" ("Transaction Step") WSVCAP_SHL_Transaction_Step_Enum."SPI Write/Read - I:SPI-Write/Read Data" ("Transaction Step") WSVCAP_SHL_Transaction_Step_Enum."RFFE Ext Write - I.Write Data" ("Transaction Step") WSVCAP_SHL_Transaction_Step_Enum."RFFE Ext Read - I:Read Data" ("Transaction Step") WSVCAP_SHL_Transaction_Step_Enum."I2C Read - I:Send Slave Address (W)" ("Transaction Step")] -> w58
              frame "I2C-Write Data" {
              }
              frame "SPI-Write/Read Data" {
              }
              frame "RFFE-Ext Write" {
              }
              frame "RFFE-Ext Read" {
              }
              frame "I2C-Read Data" {
              }
            }
            n21 = disable-structure shown="TARGET_TYPE!=FPGA" {
              disable-tunnel: w66 -> [w77 _]
              frame condition #0 (active) {
                n22 = global write "WSVCAP SHL FPGA LL RFFE Debug Global.vi" "RFFE CH (1-16)"(w77) -> ()
                n23 = global write "WSVCAP SHL FPGA LL I2C Debug Global.vi" "I2C CH (1-32)"(w77) -> ()
                n24 = global write "WSVCAP SHL FPGA LL SPI Debug Global.vi" "SPI CH (1-16)"(w77) -> ()
              }
              frame condition #1 {
              }
            }
            n25 = Multiply(x=w52, y=u8 8) -> (x*y=w50:u8)
            n26 = local write "Read Flag"(w53) -> ()
            n27 = local write "Read Status Flag"(w53) -> ()
            n28 = Bundle By Name(cluster=w69, "Wait Ticks"=w56, "Read Bits Remaining"=w50, "Transaction"=w59, "Bytes to Write"=w55, "Bytes to Read"=w52, "Sub Address"=w68, "Socket Mask"=w67, "Transaction Step"=w58, "Slave Address"=w54, "Operation Step"=WSVCAP_SHL_Operation_Step_Enum."I2C Send Slave Add - A: Send Start Sequence", "Procedure Step"=WSVCAP_SHL_Procedure_Step_Enum."I2C Start/Stop - 1: Set Clock Low", "Write CMD [1-4]"=u8 0, "Write Bit Index [0-39]"=u8 0, "Cycle Count"=u64 0 ("SPI Cycle Count"), "Wait Ticks Remaining"=u32 0, "Start Operation"=w57, "Start Procedure"=w57) -> (w70:T11)
          }
        }
      }
      frame "Pre-Transmission" {
        # "1 Second (ms)"
        # "Transfer All Data from Host into Write FIFO / Initialize Transfer State Machine and SPI Bus Data"
        n29 = disable-structure shown="TARGET_TYPE==FPGA, Default" {
          disable-tunnel: [_ i16 0] -> w78
          frame condition #0 (active) {
            n30 = property on="Waveform Chart" class="WFChart (strict)"("History Data"=cluster{i16, i16, i16, i16}[] []) -> ()  [unwired: 2 in, 2 out]
          }
          frame condition #1 {
          }
        }
        n31 = Unbundle By Name(w80) -> ("Bytes to Write"=w88:u8, "Transaction"=w81:T1)
        n32 = case shown="\"I2C-Write Data\"..\"RFFE-Ext Read\"" w81 {
          selector: w81 -> [_ w103]
          tunnel: w88 -> [_ w98]
          tunnel: [w94 w110] -> w82
          tunnel: w87 -> [w94 w109]
          tunnel: w86 -> [_ w107]
          tunnel: w85 -> [_ w106]
          tunnel: w84 -> [w93 w105]
          tunnel: [w93 w104] -> w83
          tunnel: w80 -> [w92 w100]
          tunnel: [w92 w99] -> w79
          tunnel: w78 -> [_ _]
          frame "I2C-Read Data" {
          }
          frame "I2C-Write Data".."RFFE-Ext Read" {
            # "Bits"
            # "Bytes"
            # "Not I2C"
            # "SPI/RFFE Already In Bits\nI2C Bytes to Bits"
            n33 = To Long Integer(number=w98) -> (32bit integer=w96:i32)
            n34 = Greater Or Equal?(x=w103, y=WSVCAP_SHL_Transaction_Enum."SPI-Write/Read Data" ("Transaction")) -> (x >= y?=w101:bool)
            n35 = Multiply(x=8, y=w96) -> (x*y=w97:i32)
            n36 = Select(t=w96, s=w101, f=w97) -> (s? t:f=w95:i32)
            n37 = for {
              N: w95 -> [w111]
              shift-right: [w128] -> w110
              shift-left: w109 -> [w126]
              tunnel: w103 -> [w124]
              tunnel: w107 -> [w122]
              tunnel: w106 -> [w121]
              shift-right: [w119] -> w104
              shift-left: w105 -> [w120]
              shift-right: [w113] -> w99
              shift-left: w100 -> [w114]
              i -> [w116]
              # "Fill up the FIFO/Memory with Write Data from the host"
              n38 = call "Tick Count"() -> ("Tick Count(mSec)"=w123:u32)
              n39 = flat-sequence {
                tunnel: [w137] -> w127
                tunnel: w126 -> [w138]
                tunnel: [w144] -> w125
                tunnel: w124 -> [w144]
                tunnel: w123 -> [w143]
                tunnel: w122 -> [w142]
                tunnel: w121 -> [w136]
                tunnel: w120 -> [w135]
                tunnel: [w134] -> w118
                tunnel: [w132] -> w117
                tunnel: w116 -> [w133]
                tunnel: [w131] -> w115
                tunnel: w114 -> [w131]
                tunnel: [w130] -> w112
                tunnel: w111 -> [w130]
                tunnel: [FALSE ("SPI_Write Flag")] -> w129
                tunnel: [w170] -> w128
                tunnel: w127 -> [w169]
                tunnel: w125 -> [w168]
                tunnel: [w167] -> w119
                tunnel: w118 -> [w167]
                tunnel: w117 -> [w166]
                tunnel: w115 -> [w165]
                tunnel: [w164] -> w113
                tunnel: w112 -> [w162]
                frame #0 {
                  n40 = while {
                    tunnel: w143 -> [w159]
                    tunnel: w142 -> [w157]
                    tunnel: w138 -> [w156]
                    tunnel: ["Write Flag"] -> w141
                    tunnel: [w152] -> w140
                    stop <- w154 stop-if-true
                    n41 = Unbundle By Name(w156) -> ("status"=w155:bool)
                    n42 = call "Wait"("Count(mSec)"=u32 1 ("Count(Ticks)")) -> ("Tick Count(mSec)"=w160:u32)
                    n43 = Subtract(x=w160, y=w159) -> (x-y=w158:u32)
                    n44 = Greater?(x=w158, y=w157) -> (0:w152:bool)
                    n45 = Compound Arithmetic op=OR(w155, w152, "Write Flag") -> (w154:bool)
                  }
                  n46 = To Unsigned Long Integer(number=w133) -> (unsigned 32bit integer=w132:u32)
                  n47 = Compound Arithmetic op=AND(w140, invert w141) -> (w139:bool)
                  n48 = case shown="True" w139 {
                    selector: w139 -> [_ w150]
                    tunnel: [w146 w149] -> w137
                    tunnel: w138 -> [w146 w151]
                    tunnel: w136 -> [_ w147]
                    tunnel: [w145 w147] -> w134
                    tunnel: w135 -> [w145 _]
                    frame False {
                    }
                    frame True {
                      n49 = Bundle By Name(cluster=w151, "status"=w150, "code"=9901) -> (w149:errorcluster)
                    }
                  }
                }
                frame #1 {
                  n50 = case shown="\"RFFE-Ext Write\", \"RFFE-Ext Read\"" w168 {
                    tunnel: "Write Data" -> [w172 w181 w278 _]
                    tunnel: [w175 w182 w279 w372] -> w170
                    tunnel: w169 -> [w174 w183 w280 w372]
                    tunnel: w166 -> [_ w184 w281 _]
                    tunnel: w165 -> [w173 w179 w276 w371]
                    tunnel: [w173 w180 w277 w371] -> w164
                    tunnel: w162 -> [_ w177 w274 _]
                    frame "I2C-Write Data" {
                      n51 = call "WSVCAP SHL FPGA LL I2C FIFO Manager - Pre and Post.vi"("64 Bit Data In"=w172, "error in (no error)"=w174, "Operation"=WSVCAP_SHL_FIFO_Operation_Enum."Put Element in Write") -> ("error out"=w175:errorcluster)  [unwired: 10 in, 2 out]
                    }
                    frame "SPI-Write/Read Data" {
                      # "Iteration"
                      n52 = Unbundle By Name(w179) -> ("Cycle Mode"=w178:bool)
                      n53 = case shown="Default" w184 {
                        selector: w184 -> [w186 _ _ _ _ _ _ _ _ _]
                        tunnel: w183 -> [w191 w228 w236 w241 w246 w251 w256 w261 w266 w271]
                        tunnel: [w190 w228 w236 w241 w246 w251 w256 w261 w266 w271] -> w182
                        tunnel: w181 -> [w189 w230 w235 w240 w245 w250 w255 w260 w265 w270]
                        tunnel: w179 -> [w188 w227 w238 w243 w248 w253 w258 w263 w268 w273]
                        tunnel: [w187 w229 w237 w242 w247 w252 w257 w262 w267 w272] -> w180
                        tunnel: w178 -> [w185 _ _ _ _ _ _ _ _ _]
                        tunnel: w177 -> [_ w222 _ _ _ _ _ _ _ _]
                        frame Default {
                          # "SPI Write Data"
                          n54 = case shown="False" w185 {
                            tunnel: w191 -> [w197 w199]
                            tunnel: [w196 w199] -> w190
                            tunnel: w189 -> [w192 w198]
                            tunnel: w188 -> [w193 w202]
                            tunnel: [w193 w201] -> w187
                            tunnel: w186 -> [_ w200]
                            frame False {
                              n55 = To Unsigned Word Integer(number=w192) -> (unsigned 16bit integer=w194:u16)
                              n56 = call "WSVCAP SHL FPGA LL SPI FIFO Manager - Pre and Post.vi"("Word In"=w194, "error in (no error)"=w197, "Operation"=WSVCAP_SHL_FIFO_Operation_Enum."Put Element in Write") -> ("error out"=w196:errorcluster)  [unwired: 10 in, 2 out]
                            }
                            frame True {
                              n57 = case shown="Default" w200 {
                                tunnel: [w203 w205 w208 w211 w214] -> w201
                                tunnel: w202 -> [w203 w206 w209 w212 w215]
                                tunnel: w198 -> [_ w204 w207 w210 w213]
                                frame Default {
                                }
                                frame ..9 {
                                n58 = Bundle By Name(cluster=w206, "Cycle CMD"=w204, "CMD 1"=w204) -> (w205:T11)
                                }
                                frame 10 {
                                n59 = Bundle By Name(cluster=w209, "CMD 2"=w207) -> (w208:T11)
                                }
                                frame 11 {
                                n60 = Bundle By Name(cluster=w212, "CMD 3"=w210) -> (w211:T11)
                                }
                                frame 12 {
                                n61 = Bundle By Name(cluster=w215, "CMD 4"=w213) -> (w214:T11)
                                }
                              }
                            }
                          }
                        }
                        frame 0 {
                          w223 = u8 0 ("t")
                          n62 = Unbundle By Name(w227) -> ("Bytes to Read"=w226:u8)
                          n63 = To Unsigned Long Integer(number=w230) -> (unsigned 32bit integer=w225:u32)
                          n64 = To Unsigned Byte Integer(number=w222) -> (unsigned 8bit integer=w220:u8)
                          n65 = Subtract(x=w220, y=u8 9) -> (x-y=w218:u8)
                          n66 = Quotient & Remainder(x=w218, y=u8 8) -> (floor(x/y)=w216:u8)  [unwired: 1 out]
                          n67 = Greater Than 0?(x=w225) -> (x > 0?=w224:bool)
                          n68 = Max & Min(x=w225, y=u32 1) -> (max(x,y)=w231:u32)  [unwired: 1 out]
                          n69 = Select(t=w223, s=w224, f=w226) -> ()  [unwired: 1 out]
                          n70 = Select(t=w223, s=w224, f=w216) -> (s? t:f=w219:u8)
                          n71 = To Unsigned Byte Integer(number=w231) -> (unsigned 8bit integer=w233:u8)
                          n72 = Bundle By Name(cluster=w227, "Bytes to Write"=w219, "Bytes to Read"=w219, "Cycle Mode"=w224, "Commands per Cycle [1-4]"=w233) -> (w229:T11)
                        }
                        frame 1 {
                          n73 = To Unsigned Byte Integer(number=w235) -> (unsigned 8bit integer=w234:u8)
                          n74 = Bundle By Name(cluster=w238, "CMD Length [1-48]"=w234, "CMD 1 Length (Bits)"=w234) -> (w237:T11)
                        }
                        frame 2 {
                          n75 = To Unsigned Byte Integer(number=w240) -> (unsigned 8bit integer=w239:u8)
                          n76 = Bundle By Name(cluster=w243, "CMD 2 Length (Bits)"=w239) -> (w242:T11)
                        }
                        frame 3 {
                          n77 = To Unsigned Byte Integer(number=w245) -> (unsigned 8bit integer=w244:u8)
                          n78 = Bundle By Name(cluster=w248, "CMD 3 Length (Bits)"=w244) -> (w247:T11)
                        }
                        frame 4 {
                          n79 = To Unsigned Byte Integer(number=w250) -> (unsigned 8bit integer=w249:u8)
                          n80 = Bundle By Name(cluster=w253, "CMD 4 Length (Bits)"=w249) -> (w252:T11)
                        }
                        frame 5 {
                          n81 = To Unsigned Long Integer(number=w255) -> (unsigned 32bit integer=w254:u32)
                          n82 = Bundle By Name(cluster=w258, "CMD Delay (Ticks)"=w254, "CMD 1 Delay (Ticks)"=w254) -> (w257:T11)
                        }
                        frame 6 {
                          n83 = To Unsigned Long Integer(number=w260) -> (unsigned 32bit integer=w259:u32)
                          n84 = Bundle By Name(cluster=w263, "CMD 2 Delay (Ticks)"=w259) -> (w262:T11)
                        }
                        frame 7 {
                          n85 = To Unsigned Long Integer(number=w265) -> (unsigned 32bit integer=w264:u32)
                          n86 = Bundle By Name(cluster=w268, "CMD 3 Delay (Ticks)"=w264) -> (w267:T11)
                        }
                        frame 8 {
                          n87 = To Unsigned Long Integer(number=w270) -> (unsigned 32bit integer=w269:u32)
                          n88 = Bundle By Name(cluster=w273, "CMD 4 Delay (Ticks)"=w269) -> (w272:T11)
                        }
                      }
                    }
                    frame "RFFE-Ext Write", "RFFE-Ext Read" {
                      # "Iteration"
                      n89 = Unbundle By Name(w276) -> ("Cycle Mode"=w275:bool)
                      n90 = case shown="0" w281 {
                        selector: w281 -> [w283 _ _ _ _ _ _ _ _ _]
                        tunnel: w280 -> [w288 w325 w333 w338 w343 w348 w353 w358 w363 w368]
                        tunnel: [w287 w325 w333 w338 w343 w348 w353 w358 w363 w368] -> w279
                        tunnel: w278 -> [w286 w327 w332 w337 w342 w347 w352 w357 w362 w367]
                        tunnel: w276 -> [w285 w324 w335 w340 w345 w350 w355 w360 w365 w370]
                        tunnel: [w284 w326 w334 w339 w344 w349 w354 w359 w364 w369] -> w277
                        tunnel: w275 -> [w282 _ _ _ _ _ _ _ _ _]
                        tunnel: w274 -> [_ w320 _ _ _ _ _ _ _ _]
                        frame Default {
                          # "RFFE Write Data"
                          n91 = case shown="False" w282 {
                            tunnel: w288 -> [w294 w296]
                            tunnel: [w293 w296] -> w287
                            tunnel: w286 -> [w289 w295]
                            tunnel: w285 -> [w290 w299]
                            tunnel: [w290 w298] -> w284
                            tunnel: w283 -> [_ w297]
                            frame False {
                              n92 = To Unsigned Word Integer(number=w289) -> (unsigned 16bit integer=w291:u16)
                              n93 = call "WSVCAP SHL FPGA LL RFFE FIFO Manager - Pre and Post.vi"("Word In"=w291, "error in (no error)"=w294, "Operation"=WSVCAP_SHL_FIFO_Operation_Enum."Put Element in Write") -> ("error out"=w293:errorcluster)  [unwired: 10 in, 2 out]
                            }
                            frame True {
                              n94 = case shown="..9" w297 {
                                tunnel: [w300 w302 w305 w308 w311] -> w298
                                tunnel: w299 -> [w300 w303 w306 w309 w312]
                                tunnel: w295 -> [_ w301 w304 w307 w310]
                                frame Default {
                                }
                                frame ..9 {
                                n95 = Bundle By Name(cluster=w303, "Cycle CMD"=w301, "CMD 1"=w301) -> (w302:T11)
                                }
                                frame 10 {
                                n96 = Bundle By Name(cluster=w306, "CMD 2"=w304) -> (w305:T11)
                                }
                                frame 11 {
                                n97 = Bundle By Name(cluster=w309, "CMD 3"=w307) -> (w308:T11)
                                }
                                frame 12 {
                                n98 = Bundle By Name(cluster=w312, "CMD 4"=w310) -> (w311:T11)
                                }
                              }
                            }
                          }
                        }
                        frame 0 {
                          n99 = To Unsigned Long Integer(number=w327) -> (unsigned 32bit integer=w323:u32)
                          n100 = To Unsigned Byte Integer(number=w320) -> (unsigned 8bit integer=w318:u8)
                          n101 = Subtract(x=w318, y=u8 9) -> (x-y=w316:u8)
                          n102 = Quotient & Remainder(x=w316, y=u8 8) -> (floor(x/y)=w314:u8)  [unwired: 1 out]
                          n103 = Greater Than 0?(x=w323) -> (x > 0?=w322:bool)
                          n104 = Max & Min(x=w323, y=u32 1) -> (max(x,y)=w328:u32)  [unwired: 1 out]
                          n105 = Select(t=u8 0, s=w322, f=w314) -> (s? t:f=w317:u8)
                          n106 = To Unsigned Byte Integer(number=w328) -> (unsigned 8bit integer=w330:u8)
                          n107 = Bundle By Name(cluster=w324, "Read Bytes Remaining"=u8 7, "Bytes to Write"=w317, "Cycle Mode"=w322, "Commands per Cycle [1-4]"=w330) -> (w326:T11)
                        }
                        frame 1 {
                          n108 = To Unsigned Byte Integer(number=w332) -> (unsigned 8bit integer=w331:u8)
                          n109 = Bundle By Name(cluster=w335, "CMD Length [1-48]"=w331, "CMD 1 Length (Bits)"=w331) -> (w334:T11)
                        }
                        frame 2 {
                          n110 = To Unsigned Byte Integer(number=w337) -> (unsigned 8bit integer=w336:u8)
                          n111 = Bundle By Name(cluster=w340, "CMD 2 Length (Bits)"=w336) -> (w339:T11)
                        }
                        frame 3 {
                          n112 = To Unsigned Byte Integer(number=w342) -> (unsigned 8bit integer=w341:u8)
                          n113 = Bundle By Name(cluster=w345, "CMD 3 Length (Bits)"=w341) -> (w344:T11)
                        }
                        frame 4 {
                          n114 = To Unsigned Byte Integer(number=w347) -> (unsigned 8bit integer=w346:u8)
                          n115 = Bundle By Name(cluster=w350, "CMD 4 Length (Bits)"=w346) -> (w349:T11)
                        }
                        frame 5 {
                          n116 = To Unsigned Long Integer(number=w352) -> (unsigned 32bit integer=w351:u32)
                          n117 = Bundle By Name(cluster=w355, "CMD Delay (Ticks)"=w351, "CMD 1 Delay (Ticks)"=w351) -> (w354:T11)
                        }
                        frame 6 {
                          n118 = To Unsigned Long Integer(number=w357) -> (unsigned 32bit integer=w356:u32)
                          n119 = Bundle By Name(cluster=w360, "CMD 2 Delay (Ticks)"=w356) -> (w359:T11)
                        }
                        frame 7 {
                          n120 = To Unsigned Long Integer(number=w362) -> (unsigned 32bit integer=w361:u32)
                          n121 = Bundle By Name(cluster=w365, "CMD 3 Delay (Ticks)"=w361) -> (w364:T11)
                        }
                        frame 8 {
                          n122 = To Unsigned Long Integer(number=w367) -> (unsigned 32bit integer=w366:u32)
                          n123 = Bundle By Name(cluster=w370, "CMD 4 Delay (Ticks)"=w366) -> (w369:T11)
                        }
                      }
                    }
                    frame "I2C-Read Data" {
                      # "Can't Happen"
                    }
                  }
                }
              }
              n124 = local write "Write Flag"(w129) -> ()
            }
          }
        }
      }
      frame "Transmit Data" {
        # "Perform Write/Read Operation for All Bytes"
        n125 = node-c288() -> (w379:T8)  [unwired: 1 out]
        n126 = timed-loop {
          timing-out: [_] -> w378
          timing: w379 -> [_]
          shift-right: [w405] -> w376
          shift-left: w377 -> [w413]
          tunnel: w375 -> [w410]
          tunnel: [w407] -> w374
          tunnel: [w417] -> w373
          stop <- w418 stop-if-true
          # "LD CMD"
          # "Transaction"
          # "Transaction"
          # "Transaction Finished"
          # "Procedure Finished"
          # "Next Operation Step"
          # "Operation Finished"
          # "Procedure Finished"
          # "Operation Finished"
          # "Next Operation Step"
          # "Procedure Finished"
          # "Operation Step"
          # "SPI Cycle Mode"
          # "CMD Delay (Ticks)"
          # "Transaction Step"
          n127 = call "WSVCAP SHL FPGA LL Manage Initial States.vi"("Transfer Cluster In"=w413) -> ("Transfer Cluster Out"=w411:T11)  [unwired: 14 in]
          n128 = Unbundle By Name(w411) -> ("Transaction"=w415:T1, "Transaction Step"=w414:T7, "Procedure"=w412:T12, "Bytes to Read"=w382:u8, "CMD Length [1-48]"=w390:u8, "CMD Delay (Ticks)"=w389:u32, "Start Procedure"=w400:bool, "Wait Ticks Remaining"=w399:u32, "Procedure Step"=w398:T5, "Wait Ticks"=w397:u32, "Write Bits Remaining"=w396:u8, "Write Byte"=w395:u8, "Read Bits Remaining"=w393:u8, "Read Bytes Remaining"=w381:u8, "Write Bit Index [0-39]"=w391:u8, "Cycle Mode"=w388:bool, "Cycle CMD"=w392:u64, "Socket Mask"=w394:u64, "Operation Step"=w383:T6, "Write CMD [1-4]"=w384:u8, "Commands per Cycle [1-4]"=w385:u8)
          n129 = case "Execute Procedure" shown="\"RFFE-Receive Data\"" w412 {
            tunnel: w410 -> [w620 w635 w649 w662 w673 w688 w701 w709 w725 w744 w768 w775 w788 w804 w821]
            tunnel: [w620 w634 w648 w661 w672 w687 w700 w708 w724 w743 w767 w774 w787 w803 w820] -> w409
            tunnel: [TRUE ("Finished") w633 w642 w660 w671 w682 w699 TRUE ("Finished") w712 w732 w756 TRUE ("Finished") w779 w792 w811] -> w402
            tunnel: w411 -> [w621 w630 w647 w659 w669 w686 w693 w703 w723 w736 w760 w776 w786 w802 w819]
            tunnel: [w621 w631 w646 w658 w670 w685 w692 w703 w722 w735 w759 w776 w785 w801 w818] -> w387
            tunnel: w389 -> [_ _ _ _ _ _ _ _ _ w738 w762 _ _ _ _]
            tunnel: w400 -> [_ _ _ _ _ _ _ _ _ w741 w765 _ _ _ w807]
            tunnel: w399 -> [_ w626 w644 w654 w664 w684 w696 _ w716 w740 w764 _ w782 w796 w814]
            tunnel: w398 -> [_ w628 w640 w653 w667 w678 w695 _ w717 _ _ _ w783 w797 w815]
            tunnel: w397 -> [_ w624 w639 w652 w666 w677 w694 _ w710 _ _ _ w778 w790 w809]
            tunnel: w394 -> [_ w623 w636 w650 w665 w674 w697 w704 w721 w737 w761 w773 w784 w800 w817]
            tunnel: w396 -> [_ _ w638 w651 _ _ _ _ _ _ _ _ _ _ _]
            tunnel: w395 -> [_ _ w637 _ _ _ _ _ _ _ _ _ _ _ _]
            tunnel: w393 -> [_ _ _ _ _ w676 _ _ _ _ _ _ _ _ w808]
            tunnel: w381 -> [_ _ _ _ _ w675 w689 _ _ _ _ _ _ _ w806]
            tunnel: w392 -> [_ _ _ _ _ _ _ _ w720 _ _ _ _ w799 w816]
            tunnel: w388 -> [_ _ _ _ _ _ _ _ w719 _ _ _ _ w798 _]
            tunnel: w391 -> [_ _ _ _ _ _ _ _ w718 _ _ _ _ w789 _]
            tunnel: w390 -> [_ _ _ _ _ _ _ _ w715 _ _ _ _ w795 _]
            tunnel: "Stop Cycle" -> [_ _ _ _ _ _ _ _ _ w728 w752 _ _ _ _]
            tunnel: w385 -> [_ _ _ _ _ _ _ _ _ w730 w754 _ _ _ _]
            tunnel: w384 -> [_ _ _ _ _ _ _ _ _ w727 w751 _ _ _ _]
            tunnel: w383 -> [_ w622 _ _ _ _ _ w702 _ _ _ _ _ _ _]
            tunnel: w382 -> [_ _ _ _ _ _ _ _ _ _ _ _ _ _ _]
            frame "None" {
            }
            frame "I2C-Send Start/Stop Sequence" {
              n130 = Equal?(x=w622, y=WSVCAP_SHL_Operation_Step_Enum."I2C Send Slave Add - A: Send Start Sequence" ("Operation Step")) -> (x = y?=w629:bool)
              n131 = call "WSVCAP SHL FPGA LL Procedure I2C - Send Start or Stop Sequence.vi"("Procedure Step"=w628, "Wait Ticks Remaining"=w626, "I2C Wait Ticks"=w624, "error in (no error)"=w635, "Type (T:Start; F:Stop)"=w629, "Socket Mask"=w623) -> ("Wait Ticks Remaining Out"=w625:u32, "Procedure Step Out"=w627:T5, "Finished"=w633:bool, "error out"=w634:errorcluster)  [unwired: 6 in]
              n132 = Bundle By Name(cluster=w630, "Wait Ticks Remaining"=w625, "Procedure Step"=w627) -> (w631:T11)
            }
            frame "I2C-Send Address Byte" {
              n133 = call "WSVCAP SHL FPGA LL Procedure I2C - Send Address Byte.vi"("Procedure Step"=w640, "Wait Ticks Remaining"=w644, "I2C Wait Ticks"=w639, "Write Bits Remaining"=w638, "Write Byte"=w637, "error in (no error)"=w649, "Socket Mask"=w636) -> ("Wait Ticks Remaining Out"=w643:u32, "Procedure Step Out"=w645:T5, "Write Bits Remaining Out"=w641:u8, "Finished"=w642:bool, "error out"=w648:errorcluster)  [unwired: 4 in]
              n134 = Bundle By Name(cluster=w647, "Wait Ticks Remaining"=w643, "Procedure Step"=w645, "Write Bits Remaining"=w641) -> (w646:T11)
            }
            frame "I2C-Send Data Byte" {
              n135 = call "WSVCAP SHL FPGA LL I2C Procedure - Send Data Byte.vi"("Procedure Step"=w653, "Wait Ticks Remaining"=w654, "I2C Wait Ticks"=w652, "Write Bits Remaining"=w651, "error in (no error)"=w662, "Socket Mask"=w650) -> ("Wait Ticks Remaining Out"=w657:u32, "Procedure Step Out"=w656:T5, "Write Bits Remaining Out"=w655:u8, "Finished"=w660:bool, "error out"=w661:errorcluster)  [unwired: 5 in]
              n136 = Bundle By Name(cluster=w659, "Wait Ticks Remaining"=w657, "Procedure Step"=w656, "Write Bits Remaining"=w655) -> (w658:T11)
            }
            frame "I2C-Read ACK" {
              n137 = call "WSVCAP SHL FPGA LL Procedure I2C - Read ACK.vi"("Procedure Step"=w667, "Wait Ticks Remaining"=w664, "I2C Wait Ticks"=w666, "Socket Mask"=w665, "error in (no error)"=w673) -> ("Wait Ticks Remaining Out"=w663:u32, "Procedure Step Out"=w668:T5, "Finished"=w671:bool, "error out"=w672:errorcluster)  [unwired: 6 in, 1 out]
              n138 = Bundle By Name(cluster=w669, "Wait Ticks Remaining"=w663, "Procedure Step"=w668) -> (w670:T11)
            }
            frame "I2C-Receive Byte" {
              n139 = call "WSVCAP SHL FPGA LL Procedure I2C - Receive Byte.vi"("Procedure Step"=w678, "Wait Ticks Remaining"=w684, "I2C Wait Ticks"=w677, "Read Bits Remaining"=w676, "Read Bytes Remaining"=w675, "error in (no error)"=w688, "Socket Mask"=w674) -> ("Wait Ticks Remaining Out"=w683:u32, "Procedure Step Out"=w681:T5, "Finished"=w682:bool, "Read Bits Remaining Out"=w680:u8, "Read Bytes Remaining Out"=w679:u8, "error out"=w687:errorcluster)  [unwired: 3 in]
              n140 = Bundle By Name(cluster=w686, "Wait Ticks Remaining"=w683, "Procedure Step"=w681, "Read Bits Remaining"=w680, "Read Bytes Remaining"=w679) -> (w685:T11)
            }
            frame "I2C-Write ACK" {
              n141 = Less Or Equal To 0?(x=w689) -> (x <= 0?=w698:bool)
              n142 = call "WSVCAP SHL FPGA LL Procedure I2C - Send ACK.vi"("Procedure Step"=w695, "Wait Ticks Remaining"=w696, "I2C Wait Ticks"=w694, "ACK Bit to Write"=w698, "error in (no error)"=w701, "Socket Mask"=w697) -> ("Wait Ticks Remaining Out"=w691:u32, "Procedure Step Out"=w690:T5, "Finished"=w699:bool, "error out"=w700:errorcluster)  [unwired: 6 in]
              n143 = Bundle By Name(cluster=w693, "Wait Ticks Remaining"=w691, "Procedure Step"=w690) -> (w692:T11)
            }
            frame "SPI-Clear Lines" {
              n144 = Equal?(x=w702, y=WSVCAP_SHL_Operation_Step_Enum."SPI Write/Read - A: SPI-Clear Lines") -> (x = y?=w705:bool)
              n145 = call "WSVCAP SHL FPGA LL Procedure SPI - Clear Lines.vi"("Enable SPI"=w705, "error in (no error)"=w709, "Socket Mask"=w704) -> ("error out"=w708:errorcluster)  [unwired: 12 in]
            }
            frame "SPI-Send/Receive" {
              n146 = call "WSVCAP SHL FPGA LL Procedure SPI - Send Receive.vi"("Procedure Step"=w717, "Wait Ticks Remaining"=w716, "CMD Length [1-40]"=w715, "SPI Wait Ticks"=w710, "Write Bit Index [0-39]"=w718, "SPI Cycle Mode"=w719, "error in (no error)"=w725, "SPI Cycle CMD"=w720, "Socket Mask"=w721) -> ("Wait Ticks Remaining Out"=w714:u32, "Procedure Step Out"=w713:T5, "Write Bit Index [0-39] Out"=w711:u8, "Finished"=w712:bool, "error out"=w724:errorcluster)  [unwired: 2 in]
              n147 = Bundle By Name(cluster=w723, "Wait Ticks Remaining"=w714, "Procedure Step"=w713, "Write Bit Index [0-39]"=w711) -> (w722:T11)
            }
            frame "SPI-Wait CMD Delay" {
              # "First Tick"
              # "Last Tick"
              n148 = Select(t=w738, s=w741, f=w740) -> (s? t:f=w739:u32)
              n149 = Equal?(x=w727, y=w730) -> (x = y?=w729:bool)
              n150 = Decrement(x=w739) -> (x-1=w742:u32)
              n151 = Compound Arithmetic op=AND(w729, w728) -> (w726:bool)
              n152 = Equal?(x=w739, y=w738) -> (x = y?=w734:bool)
              n153 = Less Or Equal To 0?(x=w742) -> (x <= 0?=w732:bool)
              n154 = Bundle By Name(cluster=w736, "Wait Ticks Remaining"=w742) -> (w735:T11)
              n155 = Compound Arithmetic op=AND(w732, invert w726) -> (w731:bool)
              n156 = Compound Arithmetic op=OR(w731, w734) -> (w733:bool)
              n157 = case shown="True" w733 {
                tunnel: w744 -> [w745 w749]
                tunnel: [w745 w748] -> w743
                tunnel: w737 -> [_ w747]
                tunnel: w731 -> [_ w746]
                frame False {
                }
                frame True {
                  # "First or Last Tick of Wait Cycle"
                  n158 = call "WSVCAP SHL FPGA LL Procedure SPI - Clear Lines.vi"("Enable SPI"=w746, "error in (no error)"=w749, "Socket Mask"=w747) -> ("error out"=w748:errorcluster)  [unwired: 12 in]
                }
              }
            }
            frame "RFFE-Wait CMD Delay" {
              # "First Tick"
              n159 = Select(t=w762, s=w765, f=w764) -> (s? t:f=w763:u32)
              n160 = Equal?(x=w751, y=w754) -> (x = y?=w753:bool)
              n161 = Decrement(x=w763) -> (x-1=w766:u32)
              n162 = Compound Arithmetic op=AND(w753, w752) -> (w750:bool)
              n163 = Equal?(x=w763, y=w762) -> (x = y?=w758:bool)
              n164 = Less Or Equal To 0?(x=w766) -> (x <= 0?=w756:bool)
              n165 = Bundle By Name(cluster=w760, "Wait Ticks Remaining"=w766) -> (w759:T11)
              n166 = Compound Arithmetic op=AND(w756, invert w750) -> (w755:bool)
              n167 = Compound Arithmetic op=OR(w755, w758) -> (w757:bool)
              n168 = case shown="True" w757 {
                tunnel: w768 -> [w769 w772]
                tunnel: [w769 w771] -> w767
                tunnel: w761 -> [_ w770]
                frame False {
                }
                frame True {
                  # "First or Last Tick of Wait Cycle"
                  n169 = call "WSVCAP SHL FPGA LL Procedure RFFE - Clear Lines.vi"("error in (no error)"=w772, "Socket Mask"=w770) -> ("error out"=w771:errorcluster)  [unwired: 13 in]
                }
              }
            }
            frame "RFFE-Clear Lines" {
              n170 = call "WSVCAP SHL FPGA LL Procedure RFFE - Clear Lines.vi"("error in (no error)"=w775, "Socket Mask"=w773) -> ("error out"=w774:errorcluster)  [unwired: 13 in]
            }
            frame "RFFE-Send SSC" {
              n171 = call "WSVCAP SHL FPGA LL Procedure RFFE - Send SSC.vi"("Procedure Step"=w783, "Wait Ticks Remaining"=w782, "Wait Ticks"=w778, "error in (no error)"=w788, "Socket Mask"=w784) -> ("Wait Ticks Remaining Out"=w781:u32, "Procedure Step Out"=w780:T5, "Finished"=w779:bool, "error out"=w787:errorcluster)  [unwired: 7 in]
              n172 = Bundle By Name(cluster=w786, "Wait Ticks Remaining"=w781, "Procedure Step"=w780) -> (w785:T11)
            }
            frame "RFFE-Send Data" {
              n173 = call "WSVCAP SHL FPGA LL Procedure RFFE - Send Data.vi"("Procedure Step"=w797, "Wait Ticks Remaining"=w796, "CMD Length [1-48]"=w795, "RFFE Wait Ticks"=w790, "Write Bit Index [0-47]"=w789, "RFFE Cycle Mode"=w798, "error in (no error)"=w804, "RFFE Cycle CMD"=w799, "Socket Mask"=w800) -> ("Wait Ticks Remaining Out"=w794:u32, "Procedure Step Out"=w793:T5, "Write Bit Index [0-47] Out"=w791:u8, "Finished"=w792:bool, "error out"=w803:errorcluster)  [unwired: 2 in]
              n174 = Bundle By Name(cluster=w802, "Wait Ticks Remaining"=w794, "Procedure Step"=w793, "Write Bit Index [0-39]"=w791) -> (w801:T11)
            }
            frame "RFFE-Receive Data" {
              n175 = call "WSVCAP SHL FPGA LL Procedure RFFE - Receive Data.vi"("Procedure Step"=w815, "Wait Ticks Remaining"=w814, "Start of Procedure"=w807, "RFFE Wait Ticks"=w809, "Read Bits Remaining"=w808, "Read Bytes Remaining"=w806, "error in (no error)"=w821, "RFFE Cycle CMD"=w816, "Socket Mask"=w817) -> ("Wait Ticks Remaining Out"=w813:u32, "Procedure Step Out"=w812:T5, "Read Bytes Remaining Out"=w805:u8, "Read Bits Remaining Out"=w810:u8, "Finished"=w811:bool, "error out"=w820:errorcluster)  [unwired: 1 in]
              n176 = Bundle By Name(cluster=w819, "Wait Ticks Remaining"=w813, "Procedure Step"=w812, "Read Bytes Remaining"=w805, "Read Bits Remaining"=w810) -> (w818:T11)
            }
          }
          n177 = case "Post-Procedure" shown="\"RFFE Read Data - C: Receive Byte\"" w383 {
            selector: w383 -> [w460 w463 w468 w469 w473 w477 w480 _ w487 w500 w501 w505 w507 w517 w521 w526 w528 w558 w560 w566 w571 w574 w580 w598 w614 w617]
            tunnel: [w458 w462 w466 w470 w474 w479 w482 w484 w489 w496 w503 w506 w511 w520 w523 w527 w546 w559 w562 w568 w573 w576 w582 w602 w615 w618] -> w407
            tunnel: w409 -> [w458 w462 w466 w470 w474 w479 w482 w484 w489 w497 w503 w506 w511 w520 w523 w527 w546 w559 w562 w568 w573 w576 w582 w602 w615 w618]
            tunnel: [_ _ _ w471 _ _ w481 _ _ _ w502 _ _ _ w522 _ _ _ w561 _ _ w575 _ _ _ w616] -> w401
            tunnel: w402 -> [w457 _ w465 w471 _ w476 w481 _ w485 w498 w502 _ w509 w519 w522 _ w538 w549 w561 w565 w569 w575 w578 w592 w605 w616]
            tunnel: [w456 w461 w464 w469 w472 w475 w480 WSVCAP_SHL_Operation_Step_Enum."I2C Send Data - B: Send Data Byte" ("Operation Step") w486 w499 w501 w504 w508 w518 w521 w525 w545 w557 w560 w564 w570 w574 w579 w601 w613 w617] -> w403
            tunnel: [_ _ _ _ _ _ _ _ _ _ _ _ _ _ _ TRUE ("Finished") w539 w547 _ TRUE ("Finished") _ _ TRUE ("Finished") w593 w603 _] -> w408
            tunnel: w389 -> [_ _ _ _ _ _ _ _ _ _ _ _ _ _ _ _ w535 _ _ _ _ _ _ w589 _ _]
            tunnel: w388 -> [_ _ _ _ _ _ _ _ _ _ _ _ _ _ _ _ w537 _ _ _ _ _ _ w591 _ _]
            tunnel: "Stop Cycle" -> [_ _ _ _ _ _ _ _ _ _ _ _ _ _ _ _ w531 w550 _ _ _ _ _ w585 w606 _]
            tunnel: w384 -> [_ _ _ _ _ _ _ _ _ _ _ _ _ _ _ _ w534 w552 _ _ _ _ _ w588 w608 _]
            tunnel: w385 -> [_ _ _ _ _ _ _ _ _ _ _ _ _ _ _ _ w533 w551 _ _ _ _ _ w587 w607 _]
            tunnel: w381 -> [_ _ _ _ _ _ _ _ _ _ _ _ _ w512 _ _ _ _ _ _ _ _ _ _ _ _]
            frame "I2C Send Slave Add - A: Send Start Sequence" {
              n178 = Increment(x=w460) -> (x+1=w459:T6)
              n179 = Select(t=w459, s=w457, f=w460) -> (s? t:f=w456:T6)
            }
            frame "I2C Send Slave Add - B: Load Address Byte" {
              n180 = Increment(x=w463) -> (x+1=w461:T6)
            }
            frame "I2C Send Slave Add - C: Send Address Byte" {
              n181 = Increment(x=w468) -> (x+1=w467:T6)
              n182 = Select(t=w467, s=w465, f=w468) -> (s? t:f=w464:T6)
            }
            frame "I2C Send Slave Add - D: Read Slave ACK" {
            }
            frame "I2C Send Sub Add - A: Load Sub Address" {
              n183 = Increment(x=w473) -> (x+1=w472:T6)
            }
            frame "I2C Send Sub Add - B: Send Address Byte" {
              n184 = Increment(x=w477) -> (x+1=w478:T6)
              n185 = Select(t=w478, s=w476, f=w477) -> (s? t:f=w475:T6)
            }
            frame "I2C Send Sub Add - C: Read Slave ACK" {
            }
            frame "I2C Send Data - A: Get Byte from FIFO" {
            }
            frame "I2C Send Data - B: Send Data Byte" {
              n186 = Increment(x=w487) -> (x+1=w488:T6)
              n187 = Select(t=w488, s=w485, f=w487) -> (s? t:f=w486:T6)
            }
            frame "I2C Send Data - C: Read Slave ACK" {
              n188 = call "WSVCAP SHL FPGA LL I2C FIFO Manager - Transfer.vi"("error in (no error)"=w497, "Operation"=WSVCAP_SHL_FIFO_Operation_Enum."Get Write FIFO Status") -> ("Data Out"=w494:u64, "error out"=w496:errorcluster)  [unwired: 11 in, 1 out]
              n189 = Equal To 0?(x=w494) -> (x = 0?=w493:bool)
              n190 = Select(t=WSVCAP_SHL_Operation_Step_Enum."I2C Send Data - D: Send Stop Sequence" ("Operation Step"), s=w493, f=WSVCAP_SHL_Operation_Step_Enum."I2C Send Data - A: Get Byte from FIFO" ("Operation Step")) -> (s? t:f=w490:T6)
              n191 = Select(t=w490, s=w498, f=w500) -> (s? t:f=w499:T6)
            }
            frame "I2C Send Data - D: Send Stop Sequence" {
            }
            frame "I2C Read Data - A: Load Bytes to Read" {
              n192 = Increment(x=w505) -> (x+1=w504:T6)
            }
            frame "I2C Read Data - B: Receive Byte" {
              n193 = Increment(x=w507) -> (x+1=w510:T6)
              n194 = Select(t=w510, s=w509, f=w507) -> (s? t:f=w508:T6)
            }
            frame "I2C Read Data - C: Write Master ACK" {
              n195 = Less Or Equal To 0?(x=w512) -> (x <= 0?=w513:bool)
              n196 = Increment(x=w517) -> (x+1=w515:T6)
              n197 = Select(t=w515, s=w513, f=WSVCAP_SHL_Operation_Step_Enum."I2C Read Data - B: Receive Byte" ("Operation Step")) -> (s? t:f=w514:T6)
              n198 = Select(t=w514, s=w519, f=w517) -> (s? t:f=w518:T6)
            }
            frame "I2C Read Data - D: Send Stop Sequence" {
            }
            frame "SPI Write/Read - A: SPI-Clear Lines" {
              # "Load First CMD"
              n199 = Increment(x=w526) -> (x+1=w525:T6)
            }
            frame "SPI Write/Read - B: SPI-Send/Receive Data" {
              n200 = Equal To 0?(x=w535) -> (x = 0?=w529:bool)
              n201 = Equal?(x=w534, y=w533) -> (x = y?=w532:bool)
              n202 = Compound Arithmetic op=AND(w532, w531) -> (w530:bool)
              n203 = Select(t=w528, s=w529, f=WSVCAP_SHL_Operation_Step_Enum."SPI Write/Read - C: SPI-Wait CMD Delay" ("Operation Step")) -> (s? t:f=w541:T6)
              n204 = Select(t=WSVCAP_SHL_Operation_Step_Enum."SPI Write/Read - D:SPI-Clear Lines" ("Operation Step"), s=w530, f=w541) -> (s? t:f=w540:T6)
              n205 = Select(t=w540, s=w537, f=WSVCAP_SHL_Operation_Step_Enum."SPI Write/Read - D:SPI-Clear Lines" ("Operation Step")) -> (s? t:f=w544:T6)
              n206 = Compound Arithmetic op=AND(invert w530, w529, w537, w538) -> (w539:bool)
              n207 = Select(t=w544, s=w538, f=w528) -> (s? t:f=w545:T6)
            }
            frame "SPI Write/Read - C: SPI-Wait CMD Delay" {
              n208 = Equal?(x=w552, y=w551) -> (x = y?=w553:bool)
              n209 = Compound Arithmetic op=AND(w550, w553) -> (w548:bool)
              n210 = Select(t=WSVCAP_SHL_Operation_Step_Enum."SPI Write/Read - D:SPI-Clear Lines" ("f"), s=w548, f=WSVCAP_SHL_Operation_Step_Enum."SPI Write/Read - B: SPI-Send/Receive Data") -> (s? t:f=w555:T6)
              n211 = Compound Arithmetic op=AND(invert w548, w549) -> (w547:bool)
              n212 = Select(t=w555, s=w549, f=w558) -> (s? t:f=w557:T6)
            }
            frame "SPI Write/Read - D:SPI-Clear Lines" {
            }
            frame "RFFE Read Data - A: Send SSC" {
              n213 = Increment(x=w566) -> (x+1=w567:T6)
              n214 = Select(t=w567, s=w565, f=w566) -> (s? t:f=w564:T6)
            }
            frame "RFFE Read Data - B: Send CMD Frame" {
              n215 = Increment(x=w571) -> (x+1=w572:T6)
              n216 = Select(t=w572, s=w569, f=w571) -> (s? t:f=w570:T6)
            }
            frame "RFFE Read Data - C: Receive Byte" {
            }
            frame "RFFE Write Data - A: Send SSC" {
              n217 = Increment(x=w580) -> (x+1=w581:T6)
              n218 = Select(t=w581, s=w578, f=w580) -> (s? t:f=w579:T6)
            }
            frame "RFFE Write Data - B: Send Data" {
              n219 = Equal To 0?(x=w589) -> (x = 0?=w583:bool)
              n220 = Equal?(x=w588, y=w587) -> (x = y?=w586:bool)
              n221 = Compound Arithmetic op=AND(w586, w585) -> (w584:bool)
              n222 = Select(t=WSVCAP_SHL_Operation_Step_Enum."RFFE Write Data - B: Send Data" ("Operation Step"), s=w583, f=WSVCAP_SHL_Operation_Step_Enum."RFFE Write Data - C: Wait CMD Delay" ("Operation Step")) -> (s? t:f=w595:T6)
              n223 = Select(t=WSVCAP_SHL_Operation_Step_Enum."RFFE Write Data - D: Clear Lines" ("Operation Step"), s=w584, f=w595) -> (s? t:f=w594:T6)
              n224 = Select(t=w594, s=w591, f=WSVCAP_SHL_Operation_Step_Enum."RFFE Write Data - D: Clear Lines" ("Operation Step")) -> (s? t:f=w600:T6)
              n225 = Compound Arithmetic op=AND(invert w584, w583, w591, w592) -> (w593:bool)
              n226 = Select(t=w600, s=w592, f=w598) -> (s? t:f=w601:T6)
            }
            frame "RFFE Write Data - C: Wait CMD Delay" {
              n227 = Equal?(x=w608, y=w607) -> (x = y?=w609:bool)
              n228 = Compound Arithmetic op=AND(w606, w609) -> (w604:bool)
              n229 = Select(t=WSVCAP_SHL_Operation_Step_Enum."RFFE Write Data - D: Clear Lines" ("f"), s=w604, f=WSVCAP_SHL_Operation_Step_Enum."RFFE Write Data - A: Send SSC") -> (s? t:f=w611:T6)
              n230 = Compound Arithmetic op=AND(invert w604, w605) -> (w603:bool)
              n231 = Select(t=w611, s=w605, f=w614) -> (s? t:f=w613:T6)
            }
            frame "RFFE Write Data - D: Clear Lines" {
            }
          }
          n232 = case shown="True" w408 {
            tunnel: w387 -> [w452 w455]
            tunnel: [w452 w454] -> w406
            frame False {
            }
            frame True {
              # "Load next SPI or RFFE\nCycle CMD"
              n233 = call "WSVCAP SHL FPGA LL RFFE Load Next Cycle CMD.vi"("Transfer Cluster In"=w455) -> ("Transfer Cluster Out"=w454:T11, "SPI Cycle Count"=→"Cycle Count":u64)  [unwired: 13 in]
            }
          }
          n234 = case "Post Operation" shown="\"RFFE Ext Read - I:Read Data\"" w414 {
            selector: w414 -> [w422 w426 w429 w432 w436 w440 w445 w446 w449 w451]
            tunnel: [_ _ w428 _ _ _ w444 w447 w448 w450] -> w416
            tunnel: w401 -> [w420 w424 w428 w431 w435 w439 w444 w447 w448 w450]
            tunnel: [w423 w427 w429 w430 w434 w438 w442 w446 w449 w451] -> w404
            frame "I2C Write - I:Send Slave Address" {
              n235 = Increment(x=w422) -> (x+1=w421:T7)
              n236 = Select(t=w421, s=w420, f=w422) -> (s? t:f=w423:T7)
            }
            frame "I2C Write - II:Send Sub Address" {
              n237 = Increment(x=w426) -> (x+1=w425:T7)
              n238 = Select(t=w425, s=w424, f=w426) -> (s? t:f=w427:T7)
            }
            frame "I2C Write - III:Send Data Bytes" {
            }
            frame "I2C Read - I:Send Slave Address (W)" {
              n239 = Increment(x=w432) -> (x+1=w433:T7)
              n240 = Select(t=w433, s=w431, f=w432) -> (s? t:f=w430:T7)
            }
            frame "I2C Read - II:Send Sub Address" {
              n241 = Increment(x=w436) -> (x+1=w437:T7)
              n242 = Select(t=w437, s=w435, f=w436) -> (s? t:f=w434:T7)
            }
            frame "I2C Read - III:Send Slave Address (R)" {
              n243 = Increment(x=w440) -> (x+1=w441:T7)
              n244 = Select(t=w441, s=w439, f=w440) -> (s? t:f=w438:T7)
            }
            frame "I2C Read - IV:Read Data Bytes" {
              n245 = Select(t=WSVCAP_SHL_Transaction_Step_Enum."I2C Read - I:Send Slave Address (W)" ("Transaction Step"), s=w444, f=w445) -> (s? t:f=w442:T7)
            }
            frame "SPI Write/Read - I:SPI-Write/Read Data" {
            }
            frame "RFFE Ext Write - I.Write Data" {
            }
            frame "RFFE Ext Read - I:Read Data" {
            }
          }
          n246 = Bundle By Name(cluster=w406, "Transaction Step"=w404, "Operation Step"=w403, "Start Operation"=w401, "Start Procedure"=w402) -> (w405:T11)
          n247 = disable-structure shown="TARGET_TYPE!=FPGA, default" {
            disable-tunnel: w415 -> [w822 _]
            disable-tunnel: w416 -> [_ _]
            frame condition #0 (active) {
              n248 = case shown="\"RFFE-Ext Write\", \"RFFE-Ext Read\"" w822 {
                tunnel: [w827 w840 w849] -> w823
                frame "SPI-Write/Read Data" {
                  n249 = global read "WSVCAP SHL FPGA LL SPI Debug Global.vi" "SPI_CLK"() -> (w826:bool)
                  n250 = global read "WSVCAP SHL FPGA LL SPI Debug Global.vi" "SPI_DAA"() -> (w825:bool)
                  n251 = global read "WSVCAP SHL FPGA LL SPI Debug Global.vi" "SPI_EN"() -> (w824:bool)
                  n252 = global read "WSVCAP SHL FPGA LL SPI Debug Global.vi" "SPI_DATO"() -> (w831:bool)
                  n253 = Boolean To (0,1)(Boolean=w826) -> (0, 1=w834:i16)
                  n254 = Boolean To (0,1)(Boolean=w825) -> (0, 1=w833:i16)
                  n255 = Boolean To (0,1)(Boolean=w824) -> (0, 1=w832:i16)
                  n256 = Boolean To (0,1)(Boolean=w831) -> (0, 1=w830:i16)
                  n257 = Bundle(w834, w833, w832, w830) -> (w829:cluster{i16, i16, i16, i16})  [unwired: 1 in]
                  n258 = Add(x=w829, y=cluster{i16, i16, i16, i16} {0, 2, 4, 6} ("Waveform Chart")) -> (x+y=w827:cluster{i16, i16, i16, i16})
                }
                frame "RFFE-Ext Write", "RFFE-Ext Read" {
                  n259 = global read "WSVCAP SHL FPGA LL RFFE Debug Global.vi" "RFFE_CLK"() -> (w839:bool)
                  n260 = global read "WSVCAP SHL FPGA LL RFFE Debug Global.vi" "RFFE_DAA"() -> (w838:bool)
                  n261 = global read "WSVCAP SHL FPGA LL RFFE Debug Global.vi" "RFFE_CLK"() -> (w843:bool)
                  n262 = global read "WSVCAP SHL FPGA LL RFFE Debug Global.vi" "RFFE_DATO"() -> (w836:bool)
                  n263 = Boolean To (0,1)(Boolean=w839) -> (0, 1=w845:i16)
                  n264 = Boolean To (0,1)(Boolean=w838) -> (0, 1=w844:i16)
                  n265 = Boolean To (0,1)(Boolean=w843) -> (0, 1=w837:i16)
                  n266 = Boolean To (0,1)(Boolean=w836) -> (0, 1=w835:i16)
                  n267 = Bundle(w845, w844, w837, w835) -> (w842:cluster{i16, i16, i16, i16})  [unwired: 1 in]
                  n268 = Add(x=w842, y=cluster{i16, i16, i16, i16} {0, 2, 4, 6} ("Waveform Chart")) -> (x+y=w840:cluster{i16, i16, i16, i16})
                }
                frame Default {
                  w848 = i16 0 ("0, 1")
                  n269 = global read "WSVCAP SHL FPGA LL I2C Debug Global.vi" "I2C SCL"() -> (w847:bool)
                  n270 = global read "WSVCAP SHL FPGA LL I2C Debug Global.vi" "I2C SDA"() -> (w846:bool)
                  n271 = Boolean To (0,1)(Boolean=w847) -> (0, 1=w853:i16)
                  n272 = Boolean To (0,1)(Boolean=w846) -> (0, 1=w852:i16)
                  n273 = Bundle(w853, w852, "0, 1"=w848, "0, 1"=w848) -> (w851:cluster{i16, i16, "0, 1":i16, "0, 1":i16})  [unwired: 1 in]
                  n274 = Add(x=w851, y=cluster{i16, i16, i16, i16} {0, 2, -1, -1} ("Waveform Chart")) -> (x+y=w849:cluster{i16, i16, i16, i16})
                }
              }
              "Waveform Chart" <- w823
            }
            frame condition #1 {
            }
          }
          n275 = Unbundle By Name(w407) -> ("status"=w419:bool)
          n276 = To Long Integer(number=w415) -> (32bit integer=w417:i32)
          n277 = Compound Arithmetic op=OR(w416, w419) -> (w418:bool)
        }
        n278 = node-c288(w378) -> ()
      }
      frame "Post Transmition" {
        # "1 Second (Ticks)"
        # "Error Info"
        # "Transfer Data from Read FIFO to Host"
        n279 = Unbundle By Name(w862) -> ("Bytes to Read"=w858:u8, "Transaction"=w863:T1)
        n280 = case shown="1.." w858 {
          selector: w858 -> [_ w869]
          tunnel: w865 -> [w868 w877]
          tunnel: [w868 w876] -> w864
          tunnel: w863 -> [_ w873]
          tunnel: w861 -> [_ w872]
          tunnel: [w867 w871] -> w860
          tunnel: w859 -> [w867 w870]
          frame ..0 {
            # "No Read Operation"
          }
          frame 1.. {
            # "Transfer Read Data"
            # "Read all data and transfer to the host"
            n281 = Multiply(x=w869, y=u8 8) -> (x*y=w875:u8)
            n282 = To Long Integer(number=w875) -> (32bit integer=w878:i32)
            n283 = for {
              N: w878 -> [_]
              shift-right: [w894] -> w876
              shift-left: w877 -> [w895]
              tunnel: w873 -> [w891]
              tunnel: w872 -> [w890]
              shift-right: [w881] -> w871
              shift-left: w870 -> [w879]
              i -> [w884]
              n284 = flat-sequence {
                tunnel: w895 -> [w902]
                tunnel: [w901] -> w892
                tunnel: w891 -> [w899]
                tunnel: w890 -> [w898]
                tunnel: [w898] -> w889
                tunnel: [w897] -> w885
                tunnel: w884 -> [w897]
                tunnel: [w896] -> w882
                tunnel: w879 -> [w896]
                tunnel: [w920] -> w893
                tunnel: w892 -> [w920]
                tunnel: w889 -> [w919]
                tunnel: [w919] -> w888
                tunnel: [w918] -> w886
                tunnel: w885 -> [w918]
                tunnel: [w917] -> w883
                tunnel: w882 -> [w917]
                tunnel: w893 -> [w929]
                tunnel: w888 -> [w930]
                tunnel: [w928] -> w887
                tunnel: w886 -> [w924]
                tunnel: w883 -> [w923]
                tunnel: [w922] -> w880
                tunnel: [w950] -> w894
                tunnel: w887 -> [w950]
                tunnel: [w949] -> w881
                tunnel: w880 -> [w949]
                frame #0 {
                  n285 = case shown="\"RFFE-Ext Write\", \"RFFE-Ext Read\"" w899 {
                    tunnel: w902 -> [w906 w911 w916]
                    tunnel: [w905 w910 w915] -> w901
                    tunnel: [w904 w907 w912] -> w900
                    frame "I2C-Read Data", "I2C-Write Data" {
                      n286 = call "WSVCAP SHL FPGA LL I2C FIFO Manager - Pre and Post.vi"("error in (no error)"=w906, "Operation"=WSVCAP_SHL_FIFO_Operation_Enum."Get Element from Read") -> ("64 Bit Data Out"=w904:u64, "error out"=w905:errorcluster)  [unwired: 11 in, 1 out]
                    }
                    frame "SPI-Write/Read Data" {
                      n287 = call "WSVCAP SHL FPGA LL SPI FIFO Manager - Pre and Post.vi"("error in (no error)"=w911, "Operation"=WSVCAP_SHL_FIFO_Operation_Enum."Get Element from Read") -> ("Word Out"=w909:u16, "error out"=w910:errorcluster)  [unwired: 11 in, 1 out]
                      n288 = To Unsigned Quad Integer(1:w909) -> (0:w907:u64)
                    }
                    frame "RFFE-Ext Write", "RFFE-Ext Read" {
                      n289 = call "WSVCAP SHL FPGA LL RFFE FIFO Manager - Pre and Post.vi"("error in (no error)"=w916, "Operation"=WSVCAP_SHL_FIFO_Operation_Enum."Get Element from Read") -> ("Word Out"=w914:u16, "error out"=w915:errorcluster)  [unwired: 11 in, 1 out]
                      n290 = To Unsigned Quad Integer(1:w914) -> (0:w912:u64)
                    }
                  }
                  "Read Data" <- w900
                }
                frame #1 {
                  "Read Flag" <- TRUE ("Read Flag")
                }
                frame #2 {
                  n291 = call "Tick Count2"() -> ("Tick Count(mSec)"=w931:u32)
                  n292 = while {
                    tunnel: w931 -> [w946]
                    tunnel: w930 -> [w944]
                    tunnel: w929 -> [w943]
                    tunnel: ["Ack Read"] -> w926
                    tunnel: [w940] -> w927
                    stop <- w941 stop-if-true
                    n293 = Unbundle By Name(w943) -> ("status"=w942:bool)
                    n294 = call "Wait2"("Count(mSec)"=u32 1 ("Count(Ticks)")) -> ("Tick Count(mSec)"=w947:u32)
                    n295 = Subtract(x=w947, y=w946) -> (x-y=w945:u32)
                    n296 = Greater?(x=w945, y=w944) -> (0:w940:bool)
                    n297 = Compound Arithmetic op=OR(w942, w940, "Ack Read") -> (w941:bool)
                  }
                  n298 = Compound Arithmetic op=AND(w927, invert w926) -> (w925:bool)
                  n299 = case shown="False" w925 {
                    selector: w925 -> [_ w937]
                    tunnel: [w933 w936] -> w928
                    tunnel: w929 -> [w933 w938]
                    tunnel: [w932 w934] -> w922
                    tunnel: w924 -> [_ w934]
                    tunnel: w923 -> [w932 _]
                    frame False {
                    }
                    frame True {
                      n300 = Bundle By Name(cluster=w938, "status"=w937, "code"=9902) -> (w936:errorcluster)
                    }
                  }
                }
                frame #3 {
                  n301 = local write "Ack Read"(FALSE ("Read Flag")) -> ()
                }
              }
            }
          }
        }
      }
      frame "Operation Complete" {
        # "Transfer Status"
        n302 = Unbundle By Name(w953) -> ("Cycle Mode"=w952:bool)
        n303 = To Long Integer(number=w957) -> (32bit integer=w956:i32)
        n304 = case shown="False" w952 {
          tunnel: w958 -> [w965 _]
          tunnel: w956 -> [w964 _]
          tunnel: w955 -> [w963 _]
          tunnel: w954 -> [w961 _]
          frame False {
            # "Return Status"
            n305 = for {
              N: 4 -> [_]
              tunnel: w965 -> [w972]
              tunnel: w964 -> [w971]
              tunnel: w963 -> [w970]
              tunnel: w961 -> [w966]
              i -> [w969]
              n306 = flat-sequence {
                tunnel: w972 -> [w982]
                tunnel: w971 -> [w975]
                tunnel: w970 -> [w974]
                tunnel: w969 -> [w979]
                tunnel: [w973] -> w967
                tunnel: w966 -> [w973]
                tunnel: [w987] -> w968
                tunnel: w967 -> [w987]
                tunnel: w968 -> [w989]
                frame #0 {
                  # "Iteration"
                  # "Error Info"
                  # "Last State"
                  # "Error Code"
                  # "Error Status"
                  n307 = Unbundle By Name(w982) -> ("status"=w981:bool, "code"=w976:i32)
                  n308 = Boolean To (0,1)(Boolean=w981) -> (0, 1=w980:i16)
                  n309 = To Long Integer(number=w980) -> (32bit integer=w978:i32)
                  n310 = case shown="3" w979 {
                    tunnel: [w983 w984 w985 w986] -> w977
                    tunnel: w978 -> [w983 _ _ _]
                    tunnel: w976 -> [_ w984 _ _]
                    tunnel: w975 -> [_ _ w985 _]
                    tunnel: w974 -> [_ _ _ w986]
                    frame Default {
                    }
                    frame 1 {
                    }
                    frame 2 {
                    }
                    frame 3 {
                    }
                  }
                  "Status" <- w977
                }
                frame #1 {
                  "Read Status Flag" <- TRUE ("Read Flag")
                }
                frame #2 {
                  n311 = call "Tick Count3"() -> ("Tick Count(mSec)"=w990:u32)
                  n312 = while {
                    tunnel: w990 -> [w996]
                    tunnel: w989 -> [w994]
                    stop <- w993 stop-if-true
                    n313 = call "Wait3"("Count(mSec)"=u32 1 ("Count(Ticks)")) -> ("Tick Count(mSec)"=w997:u32)
                    n314 = Subtract(x=w997, y=w996) -> (x-y=w995:u32)
                    n315 = Greater?(x=w995, y=w994) -> (0:w992:bool)
                    n316 = Compound Arithmetic op=OR(w992, "Ack Read Status") -> (w993:bool)
                  }
                }
                frame #3 {
                  n317 = local write "Ack Read Status"(FALSE ("Read Flag")) -> ()
                }
              }
            }
          }
          frame True {
            # "No Status from Cycle Mode"
          }
        }
        n318 = local write "Cmd"(WSVCAP_SHL_State."Idle" ("SPI_CMD_DBG")) -> ()
      }
    }
    n319 = Select(t=WSVCAP_SHL_Communication_Loop_State."Operation Complete" ("Action"), s=w19, f=w21) -> (s? t:f=w20:T3)
  }
  n320 = local write "Exit"(w4) -> ()
